vi "Actor Core.vi"(8 "error in":errorcluster, 11 "CS++ScopeGui.lvclass":refnum<class "CS++ScopeGui.lvclass">) -> (0 "Error Out":errorcluster, 3 "Actor out":refnum<class "Actor.lvclass">)   [LabVIEW 2015, in "CS++ScopeGui.lvlib" / "CS++ScopeGui.lvclass"]
doc: "(<B>Filename</B>: Actor Framework.lvlib:Actor.lvclass:Actor Core.vi)\n\nReceives messages to the actor, reacts to them, and initiates any error handling that may shut the actor down.\n\nDescendant classes may override this VI to append parallel tasks for the actor to complete while it handles messages. Overrides use the Call Parent Method node."
uses:
  CS++ScopeGui.lvclass
  <vilib>/ActorFramework/Actor/Actor.lvclass
  CSPP_Core/Actors/CS++BaseActor/CS++BaseActor.lvclass/CS++BaseActor.ctl
  CSPP_Core/Actors/CS++GUIActor/CS++GUIActor.lvclass/CS++GUIActor.ctl
  CSPP_Core/Classes/CS++ProcessVariables/ProcessVariable/PV.lvclass/PV.ctl
  <vilib>/ActorFramework/Actor/Actor.lvclass/Actor.ctl
  <vilib>/ActorFramework/Message Enqueuer/Message Enqueuer.lvclass/Message Enqueuer.ctl
  CSPP_Core/Actors/CS++BaseActor/Read Object Name.vi
  CSPP_Core/Actors/CS++BaseActor/Read CS++Factory.vi
  CSPP_Core/Actors/CS++GUIActor/Read Associated Actor Name.vi
  CSPP_Core/Classes/CS++ProcessVariables/ProcessVariable/Read Data.vi
  CSPP_Core/Classes/CS++ProcessVariables/ProcessVariable/Read Timestamp.vi
  CSPP_Core/Classes/CS++ProcessVariables/ProcessVariable/Read Name.vi
  CSPP_Core/Actors/CS++GUIActor/Read Stop-Event.vi
  CSPP_Core/Actors/CS++GUIActor/Read PV-Update.vi
  CSPP_Core/Actors/CS++GUIActor/Read Associated Proxy Actor Enqueuer.vi
  <vilib>/ActorFramework/Message Enqueuer/Init from Existing Queue.vi
  <vilib>/ActorFramework/Message Enqueuer/Enqueue.vi
  <vilib>/Utility/file.llb/Write To Spreadsheet File (DBL).vi
  <vilib>/ActorFramework/Message Priority Queue/Priority Enqueue.vi
  CSPP_Core/Classes/CS++ProcessVariables/PVConnection/PVConnection.lvclass
  CSPP_Core/Classes/CS++BaseClasses/Factory/CS++Factory.lvclass
  CSPP_Core/Classes/CS++ProcessVariables/ProcessVariable/PV.lvclass
  <vilib>/ActorFramework/Message Enqueuer/Message Enqueuer.lvclass
  <vilib>/ActorFramework/Stop Msg/Stop Msg.lvclass
  CSPP_Core/Actors/CS++DeviceGUIActor/CS++DeviceGUIActor.lvclass
  CSPP_Core/Libraries/Utilities/CS++Utilities.lvlib
  CSPP_Core/Actors/CS++BaseActor/CS++BaseActor.lvclass
  CSPP_Core/Actors/CS++GUIActor/CS++GUIActor.lvclass
panel:
  out "Channel Enabled?":bool[](array[boolean])
  in  "NotFirstStart":bool
  in  "OrgCurPosRight":dbl=0.4
  in  "OrgCurPosLeft":dbl=-0.4
  in  "LHS":i16=23
  in  "OrigCursPosVer":dbl[](array[numeric])=[1.25, -1.25]
  in  "DatCount":i32
  in  "Start":bool
  in  "LastModGraph":i8
  in  "Scaling-Array":dbl[](array[numeric])=[1.0, 1.0, 1.0, 1.0]
  out "LastHorOffset":dbl
  out "Complete\nData":cluster{"Array":dbl[], "Y":dbl[]}[](array[cluster])
  out "Time/Record":dbl
  out "size(s)":i32
  out "x-y":dbl
  in  "Tab Control":enum32{"Info", "Measurement"}(tab)
  out "Last Update":timestamp
  out "Associated Device Actor":string
  out "Resource Name":string
  out "Self-Test Result Message":string
  out "Self-Test Result Code":i32
  out "Firmware Revision":string
  out "Driver Revision":string
  in  "Trigger Slope":u16(ring) caption="Source" items=["Rising", "Falling"]
  in  "Trigger Source":u16(ring) caption="Source"
  in  "Trigger Level":dbl[unit] caption="Level"
  in  "One Button":bool
  in  "Abort Button":bool
  in  "RepeatButton":bool
  out "Scope Graph":cluster{dbl[], "Y":dbl[]}[](graph)
  in  "Status LED":u32(colorbox)
  in  "Config Table":string[][](table)=[["DC", "DC", "DC", "DC"], ["2", "2", "2", "2"], ["0", "0", "0", "0"], ["1", "1", "1", "1"]]
  out "Time / DIV":dbl[unit]=0.1
  in  "Horizontal Scale":i16(knob)=23 scale=0.0..31.0
  in  "Horizontal Offset":dbl[unit]
  # "Trigger"
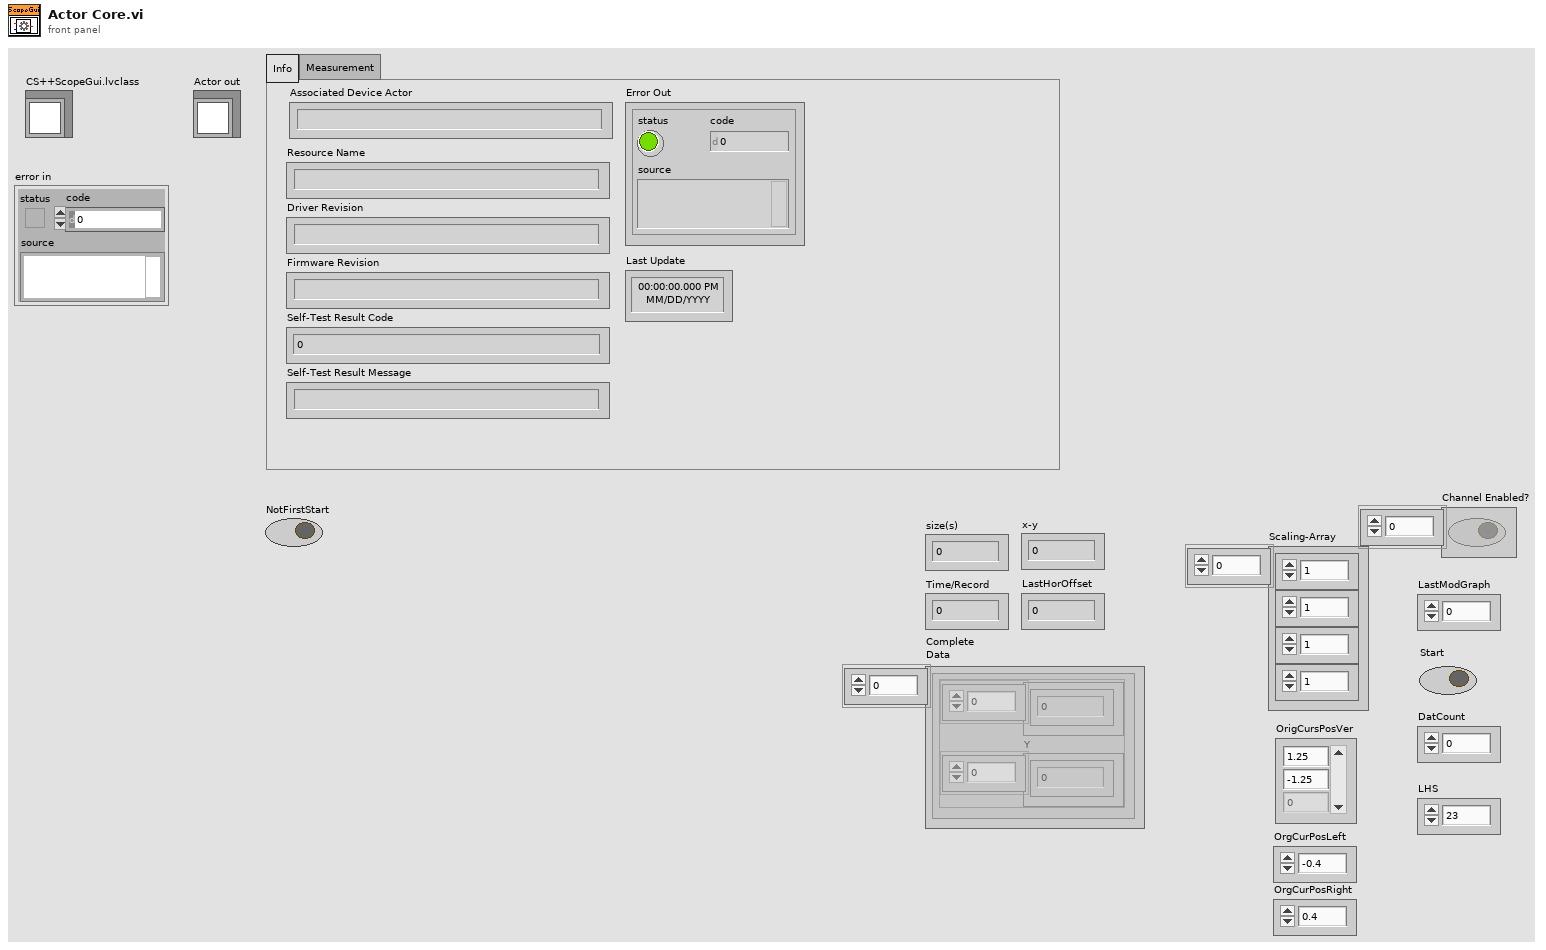
[diagram p1: front panel]
types:
  T1 = enum32{"Invalid", "Standard", "Closed", "Hidden", "Minimized", "Maximized"}
  T2 = typedef "LVAnnotationListTypeDef.ctl" = cluster{"Name":string, "Color":u32, "Style":u8, "Point Style":u8, "Name Visible":bool, "Allow Drag":bool, "Annotation Mode":u32, "Plot":i32, "Index":i32, "Position":cluster{"X":dbl, "Y":dbl}, "X Scale":u32, "Y Scale":u32, "Show Arrow":bool, "Lock Name":bool, "Plot Area":i32, "Label Offset":cluster{"X":dbl, "Y":dbl}}[]
  T3 = cluster{"Name":string, "Color":u32, "Style":u8, "Point Style":u8, "Name Visible":bool, "Allow Drag":bool, "Annotation Mode":u32, "Plot":i32, "Index":i32, "Position":cluster{"X":dbl, "Y":dbl}, "X Scale":u32, "Y Scale":u32, "Show Arrow":bool, "Lock Name":bool, "Plot Area":i32, "Label Offset":cluster{"X":dbl, "Y":dbl}}
  T4 = cluster{"Substring":string, dbl, dbl[unit], dbl[unit], bool, "vertical coupling (DC)":i32}
  T5 = cluster{dbl[unit], "min record length (100 samples)":i32, dbl[unit]}
  T6 = cluster{"Substring":string, "Trigger Level":dbl[unit], i16}
  T7 = cluster{"Substring":string, "NewVal":dbl[unit], i16}
  T8 = cluster{"Substring":string, dbl, dbl[unit], dbl[unit], "Plot.Visible?":bool, "vertical coupling (DC)":i32}
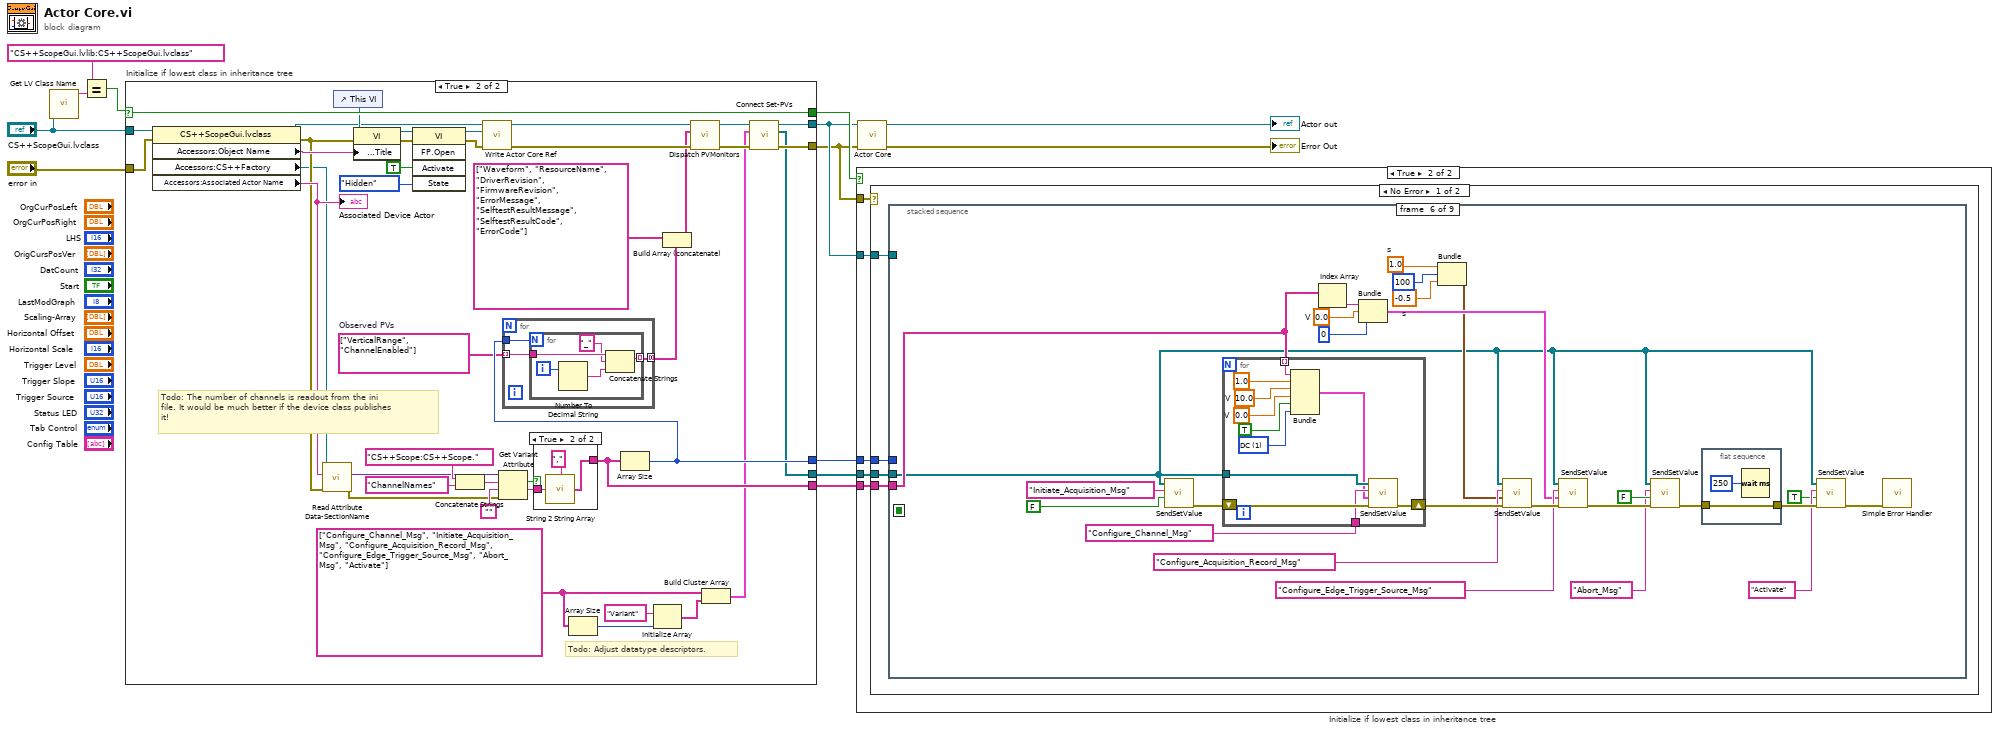
[diagram p0: block diagram]
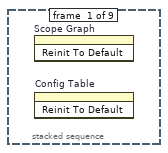
[diagram p5: hidden frame]
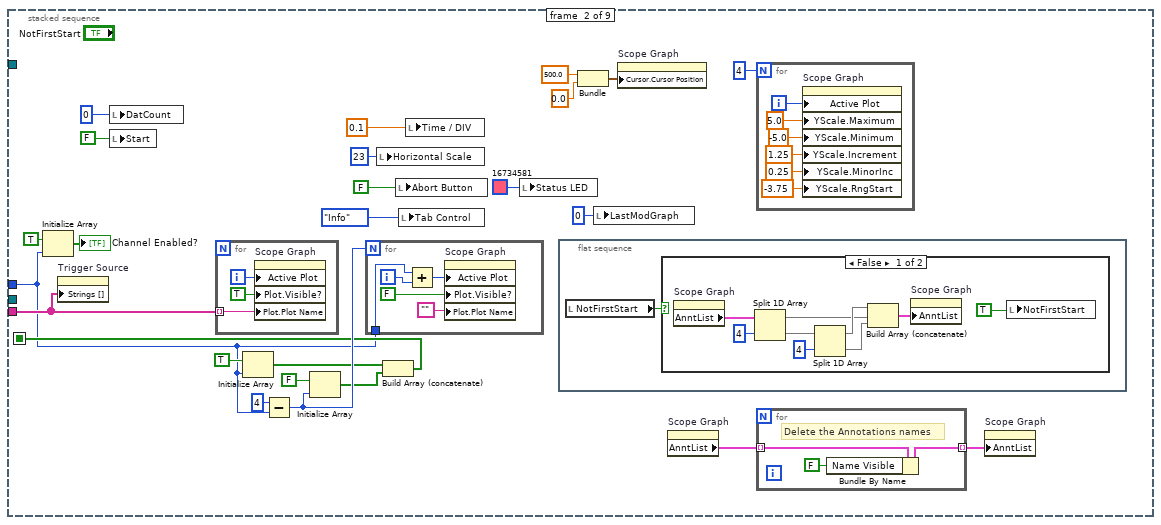
[diagram p6: hidden frame]
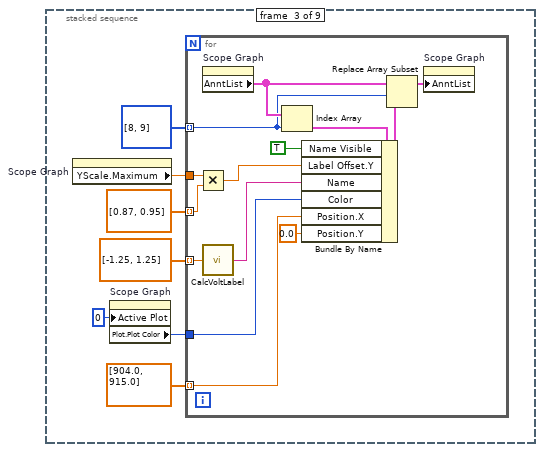
[diagram p8: hidden frame]
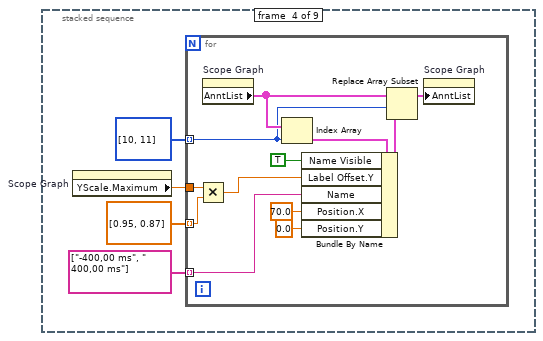
[diagram p9: hidden frame]
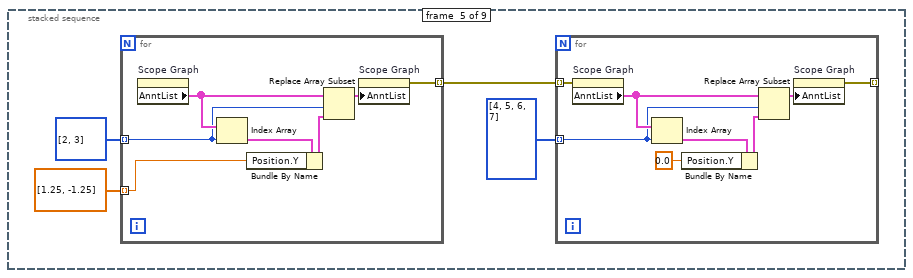
[diagram p10: hidden frame]
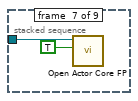
[diagram p11: hidden frame]
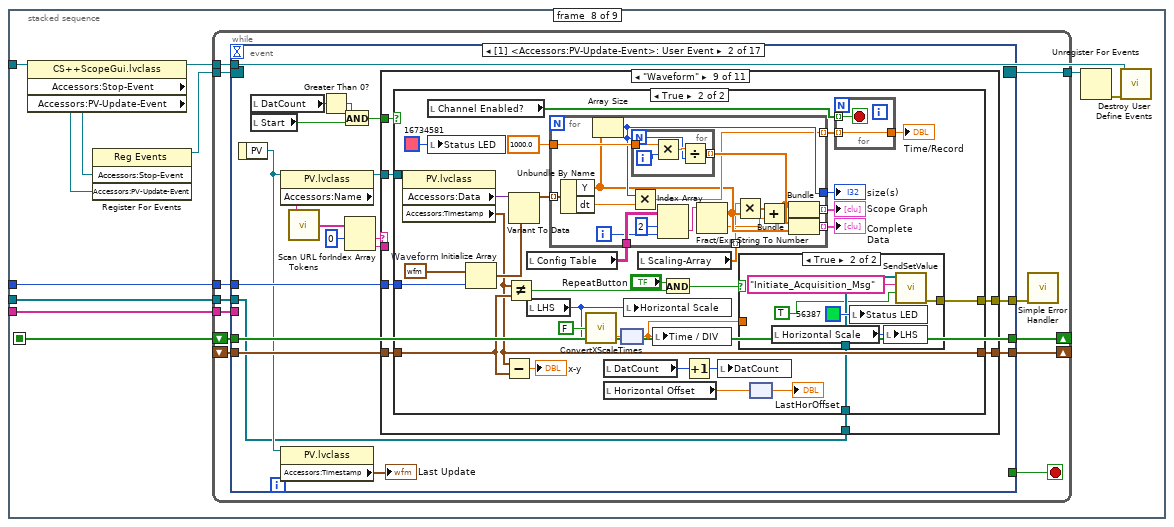
[diagram p12: hidden frame]
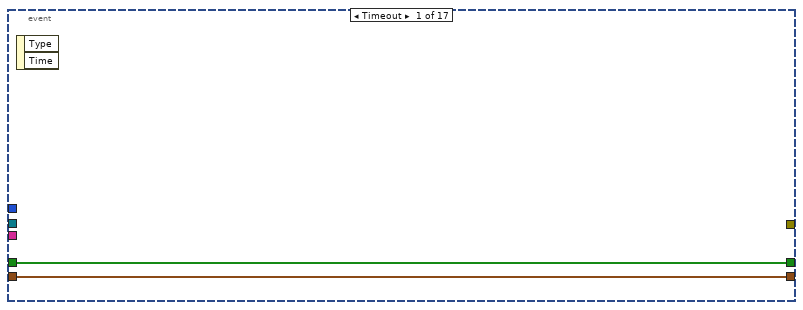
[diagram p13: hidden frame]
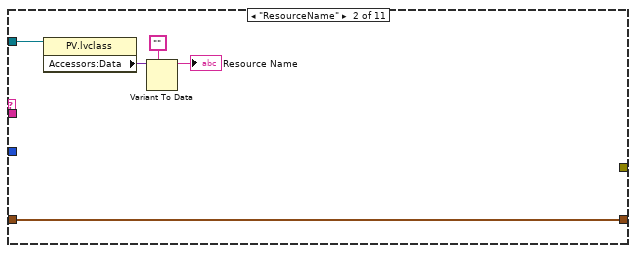
[diagram p15: hidden frame]
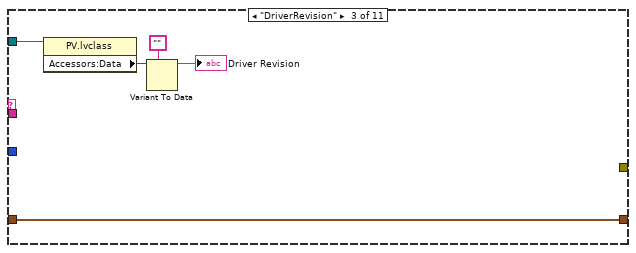
[diagram p16: hidden frame]
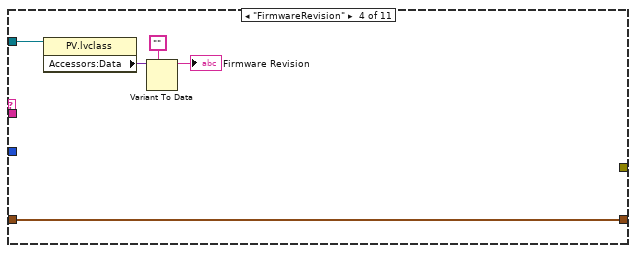
[diagram p17: hidden frame]
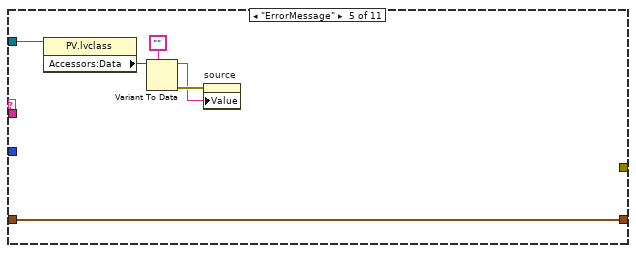
[diagram p18: hidden frame]
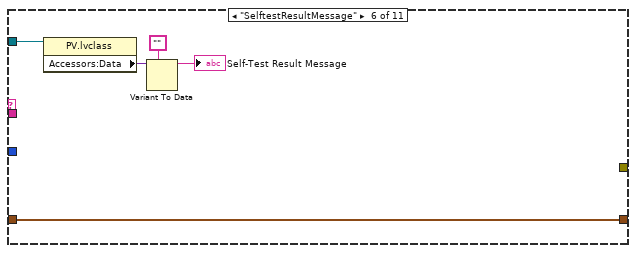
[diagram p19: hidden frame]
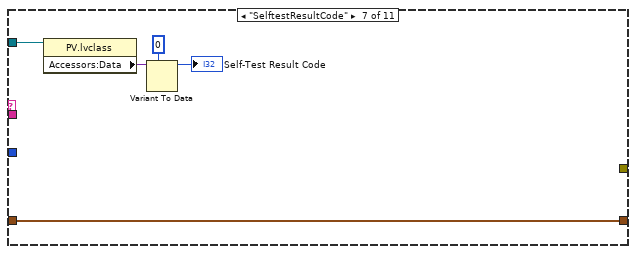
[diagram p20: hidden frame]
diagram:
  n1 = call <vilib>:"Get LV Class Name.vi"("object"="CS++ScopeGui.lvclass") -> ("class name"=w11:string)  [unwired: 9 in, 1 out]
  n2 = Equal?(x="CS++ScopeGui.lvlib:CS++ScopeGui.lvclass" ("class name"), y=w11) -> (x = y?=w9:bool)
  n3 = case "Initialize if lowest class in inheritance tree" shown="True" w9 {
    selector: w9 -> [w14 w57]
    tunnel: [w15 w24] -> w5
    tunnel: "error in" -> [w15 w37]
    tunnel: [w16 w25] -> w6
    tunnel: "CS++ScopeGui.lvclass" -> [w16 w38]
    tunnel: [w14 w57] -> w8
    tunnel: [_ w32] -> w3
    tunnel: [_ w50] -> w2
    tunnel: [_ w22] -> w1
    frame False {
    }
    frame True {
      w21 = string[] ["Configure_Channel_Msg", "Initiate_Acquisition_Msg", "Configure_Acquisition_Record_Msg", "Configure_Edge_Trigger_Source_Msg", "Abort_Msg", "Activate"]
      w31 = string[] ["VerticalRange", "ChannelEnabled"]  # Observed PVs
      # "Todo: Adjust datatype descriptors."
      # "Todo: The number of channels is readout from the ini\nfile. It would be much better if the device class publishes\nit!"
      n4 = property class="CS++ScopeGui.lvclass"(reference=w38, error in=w37) -> (reference out=w42:refnum<class "CS++ScopeGui.lvclass">, error out=w35:errorcluster, "Accessors:Object Name"=w41:string, "Accessors:CS++Factory"=w27:refnum<class "CS++Factory.lvclass">, "Accessors:Associated Actor Name"=w36:string)
      "Associated Device Actor" <- w36
      n5 = call-dynamic "Read Attribute Data-SectionName.vi"("error in (no error)"=w35, "Object Name"=w36, "CS++Factory in"=w27) -> ("error out"=w33:errorcluster, "Attribute Data"=w34:variant)  [unwired: 6 in, 1 out]
      n6 = control-ref of="This VI"() -> (w45:refnum<vi>)
      n7 = property class="VI"(reference=w45, error in=w35, "Front Panel.Title"=w41) -> (reference out=w44:refnum<vi>, error out=w43:errorcluster)
      n8 = invoke class="VI" method="FP.Open"(reference=w44, error in=w43, "Activate"=TRUE ("Activate?"), "State"=T1."Hidden") -> (reference out=w47:refnum<vi>, error out=w46:errorcluster)  [unwired: 1 in, 3 out]
      n9 = Concatenate Strings("CS++Scope:CS++Scope.", "ChannelNames" ("string")) -> (w55:string)
      n10 = call "Write Actor Core Ref.vi"("error in (no error)"=w46, "Actor Core Ref"=w47, "CS++BaseActor in"=w42) -> ("error out"=w39:errorcluster, "CS++BaseActor out"=w40:refnum<class "CS++ScopeGui.lvclass">)  [unwired: 7 in]
      n11 = Get Variant Attribute(Variant=w34, name=w55, default value (empty Variant)="", error in=w33) -> (found=w52:bool, value=w53:string)  [unwired: 2 out]
      n12 = case shown="True" w52 {
        tunnel: w53 -> [_ w68]
        tunnel: [_ w66] -> w50
        frame False {
        }
        frame True {
          n13 = call "String 2 String Array.vi"("String"=w68, "Delimiter (\",\")"="," ("Delimiter (\",\")")) -> ("Substrings"=w66:string[])
        }
      }
      n14 = Array Size(array=w21) -> (size(s)=w20:i32)
      n15 = Array Size(array=w50) -> (size(s)=w32:i32)
      n16 = for {
        tunnel: w32 -> [w60]
        tunnel: w31 -> [w59] mode=indexing
        tunnel: [w58] -> w30 mode=concatenating
        n17 = for {
          N: w60 -> [_]
          tunnel: w59 -> [w65]
          tunnel: [w64] -> w58 mode=indexing
          i -> [w63]
          n18 = Number To Decimal String(number=w63) -> (decimal integer string=w62:string)  [unwired: 1 in]
          n19 = Concatenate Strings(w65, "_" ("string"), w62) -> (w64:string)
        }
      }
      n20 = Initialize Array("Variant", w20) -> (w17:string[])
      n21 = Build Array (concatenate)(string[] ["Waveform", "ResourceName", "DriverRevision", "FirmwareRevision", "ErrorMessage", "SelftestResultMessage", "SelftestResultCode", "ErrorCode"], w30) -> (w29:string[])
      n22 = call "Dispatch PVMonitors.vi"("Error In"=w39, "PV Names (empty)"=w29, "CS++GUIActor in"=w40) -> ("Error Out"=w23:errorcluster, "CS++GUIActor out"=w26:refnum<class "CS++ScopeGui.lvclass">)  [unwired: 7 in]
      n23 = Build Cluster Array(w21, w17) -> (w18:cluster{string, string}[])
      n24 = call "Connect Set-PVs.vi"("Error In"=w23, "Set-Messages"=w18, "CS++GUIActor in"=w26) -> ("Error Out"=w24:errorcluster, "PVConnections"=w22:refnum<class "PVConnection.lvclass">[], "CS++GUIActor out"=w25:refnum<class "CS++ScopeGui.lvclass">)  [unwired: 6 in]
    }
  }
  n25 = case "Initialize if lowest class in inheritance tree" shown="True" w8 {
    tunnel: w5 -> [_ w73]
    tunnel: w6 -> [_ w72]
    tunnel: w3 -> [_ w71]
    tunnel: w2 -> [_ w70]
    tunnel: w1 -> [_ w69]
    frame False {
    }
    frame True {
      n26 = case shown="No Error" w73 {
        tunnel: w72 -> [w77 _]
        tunnel: w71 -> [w76 _]
        tunnel: w70 -> [w75 _]
        tunnel: w69 -> [w74 _]
        frame No Error {
          n27 = stacked-sequence {
            seq-local: [_ w86 _ _ _ _ _ _ _] -> [_ _ _ _ _ _ _ w235 _]
            tunnel: w77 -> [_ _ _ _ _ _ w225 w232 w1117]
            tunnel: w76 -> [_ w79 _ _ _ _ _ w237 _]
            tunnel: w75 -> [_ w93 _ _ _ w200 _ w236 _]
            tunnel: w74 -> [_ _ _ _ _ w188 _ w227 w1115]
            frame #0 {
              n28 = invoke on="Scope Graph" class="XYGraph (strict)" method="Reinit To Default"() -> ()  [unwired: 3 in, 3 out]
              n29 = invoke on="Config Table" class="Tbl (strict)" method="Reinit To Default"() -> ()  [unwired: 3 in, 3 out]
            }
            frame #1 {
              n30 = Initialize Array(TRUE ("Open FP (F)"), w79) -> (→"Channel Enabled?":bool[])
              n31 = property on="Trigger Source" class="Ring (strict)"("Strings []"=w93) -> ()  [unwired: 2 in, 2 out]
              n32 = local write "DatCount"(0 ("DataCounter")) -> ()
              n33 = local write "Start"(FALSE ("Start")) -> ()
              n34 = for {
                tunnel: w93 -> [w127] mode=indexing
                i -> [w129]
                n35 = property on="Scope Graph" class="XYGraph (strict)"("Active Plot"=w129, "Plot.Visible?"=TRUE ("Plot.Visible"), "Plot.Plot Name"=w127) -> ()  [unwired: 2 in, 2 out]
              }
              n36 = Initialize Array(TRUE ("Plot.Visible?"), w79) -> (w88:bool[])
              n37 = Subtract(x=4, y=w79) -> (x-y=w89:i32)
              n38 = Initialize Array(FALSE ("Plot.Visible?"), w89) -> (w87:bool[])
              n39 = for {
                N: w89 -> [_]
                tunnel: w79 -> [w120]
                i -> [w122]
                n40 = Add(x=w120, y=w122) -> (x+y=w121:i32)
                n41 = property on="Scope Graph" class="XYGraph (strict)"("Active Plot"=w121, "Plot.Visible?"=FALSE ("Plot.Visible"), "Plot.Plot Name"="") -> ()  [unwired: 2 in, 2 out]
              }
              n42 = local write "Horizontal Scale"(i16 23 ("Horizontal Scale")) -> ()
              n43 = Build Array (concatenate)(w88, w87) -> (w86:bool[])
              n44 = local write "Abort Button"(FALSE ("Stop Button")) -> ()
              n45 = local write "Tab Control"(enum32{"Info", "Measurement"}."Info" ("Tab Control")) -> ()
              n46 = local write "Time / DIV"(dbl[unit] 0.1 ("Time / DIV")) -> ()
              n47 = local write "Status LED"(u32 16734581) -> ()
              n48 = flat-sequence {
                frame #0 {
                  n49 = local read "NotFirstStart"() -> (w103:bool)
                  n50 = case shown="False" w103 {
                    frame False {
                      n51 = property on="Scope Graph" class="XYGraph (strict)"() -> ("AnntList"=w112:T2)  [unwired: 2 in, 2 out]
                      n52 = Split 1D Array(array=w112, index=4) -> (first subarray=w107:T2, second subarray=w110:T2)
                      n53 = Split 1D Array(array=w110, index=4) -> (first subarray=w108:T2, second subarray=w106:T2)
                      n54 = Build Array (concatenate)(w108, w107, w106) -> (w105:T2)
                      n55 = property on="Scope Graph" class="XYGraph (strict)"("AnntList"=w105) -> ()  [unwired: 2 in, 2 out]
                      n56 = local write "NotFirstStart"(TRUE ("FirstStart")) -> ()
                    }
                    frame True {
                    }
                  }
                }
              }
              n57 = Bundle(500.0, 0.0) -> (w94:cluster{dbl, dbl})  [unwired: 1 in]
              n58 = local write "LastModGraph"(u8 0 ("LastModifiedGraph")) -> ()
              n59 = property on="Scope Graph" class="XYGraph (strict)"("Cursor.Cursor Position"=w94) -> ()  [unwired: 2 in, 2 out]
              n60 = property on="Scope Graph" class="XYGraph (strict)"() -> ("AnntList"=w100:T2)  [unwired: 2 in, 2 out]
              n61 = for {
                N: 4 -> [_]
                i -> [w118]
                n62 = property on="Scope Graph" class="XYGraph (strict)"("Active Plot"=w118, "YScale.Maximum"=5.0, "YScale.Minimum"=-5.0 ("Y Scale.Range:Minimum"), "YScale.Increment"=1.25 ("Y Scale.Range:Increment"), "YScale.MinorInc"=0.25 ("Y Scale.Range:Minor Increment"), "YScale.RngStart"=-3.75 ("Y Scale.Range:Start")) -> ()  [unwired: 2 in, 2 out]
              }
              n63 = for {
                tunnel: w100 -> [w125] mode=indexing
                tunnel: [w124] -> w99 mode=indexing
                # "Delete the Annotations names"
                n64 = Bundle By Name(cluster=w125, "Name Visible"=FALSE) -> (w124:T3)
              }
              n65 = property on="Scope Graph" class="XYGraph (strict)"("AnntList"=w99) -> ()  [unwired: 2 in, 2 out]
            }
            frame #2 {
              n66 = property on="Scope Graph" class="XYGraph (strict)"() -> ("YScale.Maximum"=w135:dbl)  [unwired: 2 in, 2 out]
              n67 = property on="Scope Graph" class="XYGraph (strict)"("Active Plot"=u32 0) -> ("Plot.Plot Color"=w132:u32)  [unwired: 2 in, 2 out]
              n68 = for {
                tunnel: i32[] [8, 9] -> [w145] mode=indexing
                tunnel: w135 -> [w143]
                tunnel: dbl[] [0.87, 0.95] -> [w142] mode=indexing
                tunnel: dbl[] [-1.25, 1.25] -> [w138] mode=indexing
                tunnel: w132 -> [w141]
                tunnel: dbl[] [904.0, 915.0] -> [w140] mode=indexing
                n69 = Multiply(x=w143, y=w142) -> (x*y=w144:dbl)
                n70 = property on="Scope Graph" class="XYGraph (strict)"() -> ("AnntList"=w149:T2)  [unwired: 2 in, 2 out]
                n71 = call "CalcVoltLabel.vi"("InputVolt"=w138) -> ("VoltString"=w137:string)
                n72 = Index Array(array=w149, index=w145) -> (element=w148:T3)
                n73 = Bundle By Name(cluster=w148, "Name Visible"=TRUE, "Label Offset.Y"=w144, "Name"=w137, "Color"=w141, "Position.X"=w140, "Position.Y"=0.0) -> (w147:T3)
                n74 = Replace Array Subset(array=w149, new element=w147, index=w145) -> (w150:T2)
                n75 = property on="Scope Graph" class="XYGraph (strict)"("AnntList"=w150) -> ()  [unwired: 2 in, 2 out]
              }
            }
            frame #3 {
              n76 = property on="Scope Graph" class="XYGraph (strict)"() -> ("YScale.Maximum"=w153:dbl)  [unwired: 2 in, 2 out]
              n77 = for {
                tunnel: i32[] [10, 11] -> [w161] mode=indexing
                tunnel: w153 -> [w159]
                tunnel: dbl[] [0.95, 0.87] -> [w158] mode=indexing
                tunnel: string[] ["-400,00 ms", " 400,00 ms"] -> [w157] mode=indexing
                n78 = Multiply(x=w159, y=w158) -> (x*y=w160:dbl)
                n79 = property on="Scope Graph" class="XYGraph (strict)"() -> ("AnntList"=w165:T2)  [unwired: 2 in, 2 out]
                n80 = Index Array(array=w165, index=w161) -> (element=w164:T3)
                n81 = Bundle By Name(cluster=w164, "Name Visible"=TRUE, "Label Offset.Y"=w160, "Name"=w157, "Position.X"=70.0, "Position.Y"=0.0) -> (w163:T3)
                n82 = Replace Array Subset(array=w165, new element=w163, index=w161) -> (w166:T2)
                n83 = property on="Scope Graph" class="XYGraph (strict)"("AnntList"=w166) -> ()  [unwired: 2 in, 2 out]
              }
            }
            frame #4 {
              n84 = for {
                tunnel: i32[] [2, 3] -> [w181] mode=indexing
                tunnel: dbl[] [1.25, -1.25] -> [w180] mode=indexing
                tunnel: [w179] -> w168 mode=indexing
                n85 = property on="Scope Graph" class="XYGraph (strict)"() -> ("AnntList"=w184:T2)  [unwired: 2 in, 2 out]
                n86 = Index Array(array=w184, index=w181) -> (element=w183:T3)
                n87 = Bundle By Name(cluster=w183, "Position.Y"=w180) -> (w182:T3)
                n88 = Replace Array Subset(array=w184, new element=w182, index=w181) -> (w185:T2)
                n89 = property on="Scope Graph" class="XYGraph (strict)"("AnntList"=w185) -> (error out=w179:errorcluster)  [unwired: 2 in, 1 out]
              }
              n90 = for {
                tunnel: i32[] [4, 5, 6, 7] -> [w174] mode=indexing
                tunnel: [w173] -> _ mode=indexing
                tunnel: w168 -> [w172] mode=indexing
                n91 = property on="Scope Graph" class="XYGraph (strict)"(error in=w172) -> ("AnntList"=w177:T2)  [unwired: 1 in, 2 out]
                n92 = Index Array(array=w177, index=w174) -> (element=w176:T3)
                n93 = Bundle By Name(cluster=w176, "Position.Y"=0.0) -> (w175:T3)
                n94 = Replace Array Subset(array=w177, new element=w175, index=w174) -> (w178:T2)
                n95 = property on="Scope Graph" class="XYGraph (strict)"("AnntList"=w178) -> (error out=w173:errorcluster)  [unwired: 2 in, 1 out]
              }
            }
            frame #5 {
              w196 = dbl[unit] -0.5  # s
              w198 = dbl[unit] 1.0  # s
              w202 = dbl[unit] 0.0  # V
              n96 = call "SendSetValue.vi"("Data"=FALSE, "PVName"="Initiate_Acquisition_Msg", "PVConnections"=w188) -> ("error out"=w209:errorcluster)  [unwired: 7 in, 1 out]
              n97 = for {
                tunnel: w188 -> [w222]
                tunnel: "Configure_Channel_Msg" -> [w221]
                shift-right: [w223] -> w208
                shift-left: w209 -> [w224]
                tunnel: w200 -> [w217] mode=indexing
                w214 = dbl[unit] 0.0  # V
                w215 = dbl[unit] 10.0  # V
                w220 = 1 items=["AC", "DC", "GND"] ("vertical coupling (DC)")
                n98 = Bundle("Substring"=w217, 1.0, w215, w214, TRUE, "vertical coupling (DC)"=w220) -> (w218:T4)  [unwired: 1 in]
                n99 = call "SendSetValue.vi"("error in (no error)"=w224, "Data"=w218, "PVName"=w221, "PVConnections"=w222) -> ("error out"=w223:errorcluster)  [unwired: 6 in, 1 out]
              }
              n100 = Index Array(array=w200) -> (element=w201:string)  [unwired: 1 in]
              n101 = Bundle("Substring"=w201, w202, i16 0) -> (w199:cluster{"Substring":string, dbl[unit], i16})  [unwired: 1 in]
              n102 = Bundle(w198, "min record length (100 samples)"=100, w196) -> (w197:T5)  [unwired: 1 in]
              n103 = call "SendSetValue.vi"("error in (no error)"=w208, "Data"=w197, "PVName"="Configure_Acquisition_Record_Msg", "PVConnections"=w188) -> ("error out"=w207:errorcluster)  [unwired: 6 in, 1 out]
              n104 = call "SendSetValue.vi"("error in (no error)"=w207, "Data"=w199, "PVName"="Configure_Edge_Trigger_Source_Msg", "PVConnections"=w188) -> ("error out"=w190:errorcluster)  [unwired: 6 in, 1 out]
              n105 = call "SendSetValue.vi"("error in (no error)"=w190, "Data"=FALSE, "PVName"="Abort_Msg", "PVConnections"=w188) -> ("error out"=w189:errorcluster)  [unwired: 6 in, 1 out]
              n106 = flat-sequence {
                tunnel: [w213] -> w193
                tunnel: w189 -> [w213]
                frame #0 {
                  n107 = Wait (ms)(milliseconds to wait=u32 250) -> ()  [unwired: 1 out]
                }
              }
              n108 = call "SendSetValue.vi"("error in (no error)"=w193, "Data"=TRUE, "PVName"="Activate", "PVConnections"=w188) -> ("error out"=w194:errorcluster)  [unwired: 6 in, 1 out]
              n109 = call <vilib>:"Simple Error Handler.vi"("error in (no error)"=w194) -> ()  [unwired: 4 in, 5 out]
            }
            frame #6 {
              n110 = call "Open Actor Core FP.vi"("Open FP (F)"=TRUE, "CS++BaseActor in"=w225) -> ()  [unwired: 8 in, 2 out]
            }
            frame #7 {
              n111 = property class="CS++ScopeGui.lvclass"(reference=w232) -> (reference out=w231:refnum<class "CS++ScopeGui.lvclass">, "Accessors:Stop-Event"=w229:refnum<user-event>, "Accessors:PV-Update-Event"=w228:refnum<user-event>)  [unwired: 1 in, 1 out]
              n112 = register-events(w229, w228) -> (reference out=w230:refnum<event-registration>)  [unwired: 2 in, 1 out]
              n113 = while {
                tunnel: w230 -> [w249]
                tunnel: w231 -> [w248]
                tunnel: [w246] -> w234
                tunnel: w237 -> [w244]
                shift-right: [w243] -> _
                shift-left: _ -> [w242]
                tunnel: w236 -> [w241]
                shift-right: [w240] -> _
                shift-left: w235 -> [w239]
                tunnel: w227 -> [w238]
                stop <- w247 stop-if-true
                n114 = event shown="[1] <Accessors:PV-Update-Event>: User Event" {
                  selector: w249 -> [_ _ _ _ _ _ _ _ _ _ _ _ _ _ _ _ _]
                  dyn-events: [_ _ _ _ _ _ _ _ _ _ _ _ _ _ _ _ _] -> w246
                  timeout: _ -> [_ _ _ _ _ _ _ _ _ _ _ _ _ _ _ _ _]
                  tunnel: w248 -> [_ _ _ _ _ _ _ _ _ _ _ _ _ _ _ _ w1109]
                  tunnel: [_ _ _ _ _ _ _ _ _ _ _ _ _ w1067 w1094 _ _] -> w247
                  tunnel: [_ w266 _ _ _ _ _ w632 w758 w770 w804 _ _ _ _ w1097 _] -> w245
                  tunnel: w244 -> [_ w265 _ _ _ _ _ w624 _ _ w781 _ _ w1066 _ _ _]
                  tunnel: [w251 w264 w482 w555 w594 w606 w618 w634 w757 w769 w806 w943 w1064 w1069 w1095 w1100 w1108] -> w243
                  tunnel: w242 -> [w251 w263 w482 w555 w594 w606 w618 w634 w757 w769 w806 w943 w1064 w1069 w1095 w1100 w1108]
                  tunnel: w241 -> [_ _ _ _ w597 w609 w621 w631 _ _ w803 _ _ _ _ _ _]
                  tunnel: [w250 w261 w483 w556 w595 w607 w619 w623 w756 w768 w783 w940 w1065 w1070 w1093 w1099 w1106] -> w240
                  tunnel: w239 -> [w250 w261 w483 w556 w595 w607 w619 w626 w756 w768 w783 w940 w1065 w1070 w1093 w1099 w1106]
                  tunnel: w238 -> [_ w252 w442 w518 w587 w599 w611 w622 w755 w767 w780 _ _ _ _ w1098 _]
                  event Timeout {
                    n115 = event-data() -> ()  [unwired: 1 in, 2 out]
                  }
                  event User Event {
                    n116 = event-data() -> ("PV"=w254:refnum<class "PV.lvclass">)  [unwired: 1 in]
                    n117 = local read "DatCount"() -> (w260:i32)
                    n118 = local read "Start"() -> (w258:bool)
                    n119 = property class="PV.lvclass"(reference=w254) -> (reference out=w256:refnum<class "PV.lvclass">, "Accessors:Name"=w255:string)  [unwired: 1 in, 1 out]
                    n120 = property class="PV.lvclass"(reference=w254) -> ("Accessors:Timestamp"=→"Last Update":timestamp)  [unwired: 1 in, 2 out]
                    n121 = call "Scan URL for Tokens.vi"("URL"=w255) -> ("Tokens"=w268:string[])
                    n122 = Greater Than 0?(x=w260) -> (x > 0?=w259:bool)
                    n123 = And(x=w259, y=w258) -> (x .and. y?=w257:bool)
                    n124 = Index Array(array=w268, index #1=0 ("index")) -> (element #1=w267:string, element #2=w262:string)  [unwired: 1 in]
                    n125 = case shown="\"Waveform\"" w267 {
                      tunnel: w256 -> [_ w273 w278 w283 w289 w294 w299 w305 w314 w411 w420]
                      tunnel: [_ _ _ _ _ _ _ _ w313 _ _] -> w266
                      tunnel: w265 -> [_ _ _ _ _ _ _ _ w312 w380 _]
                      tunnel: [w270 w271 w276 w281 w286 w292 w297 w302 w310 w410 w419] -> w264
                      tunnel: w263 -> [w270 w271 w276 w281 w286 w292 w297 w302 w311 w410 w419]
                      tunnel: w262 -> [_ _ _ _ _ _ _ _ _ w395 w418]
                      tunnel: w257 -> [_ _ _ _ _ _ _ _ w309 _ _]
                      tunnel: w252 -> [_ _ _ _ _ _ _ _ w308 _ _]
                      frame Default {
                      }
                      frame "ResourceName" {
                        n126 = property class="PV.lvclass"(reference=w273) -> ("Accessors:Data"=w275:variant)  [unwired: 1 in, 2 out]
                        n127 = Variant To Data(type="", Variant=w275) -> (data=→"Resource Name":string)  [unwired: 1 in, 1 out]
                      }
                      frame "DriverRevision" {
                        n128 = property class="PV.lvclass"(reference=w278) -> ("Accessors:Data"=w280:variant)  [unwired: 1 in, 2 out]
                        n129 = Variant To Data(type="", Variant=w280) -> (data=→"Driver Revision":string)  [unwired: 1 in, 1 out]
                      }
                      frame "FirmwareRevision" {
                        n130 = property class="PV.lvclass"(reference=w283) -> ("Accessors:Data"=w285:variant)  [unwired: 1 in, 2 out]
                        n131 = Variant To Data(type="", Variant=w285) -> (data=→"Firmware Revision":string)  [unwired: 1 in, 1 out]
                      }
                      frame "ErrorMessage" {
                        n132 = property class="PV.lvclass"(reference=w289) -> ("Accessors:Data"=w291:variant)  [unwired: 1 in, 2 out]
                        n133 = Variant To Data(type="", Variant=w291) -> (data=w287:string, error out=w288:errorcluster)  [unwired: 1 in]
                        n134 = property on="source" class="Str"(error in=w288, "Value"=w287) -> ()  [unwired: 1 in, 2 out]
                      }
                      frame "SelftestResultMessage" {
                        n135 = property class="PV.lvclass"(reference=w294) -> ("Accessors:Data"=w296:variant)  [unwired: 1 in, 2 out]
                        n136 = Variant To Data(type="", Variant=w296) -> (data=→"Self-Test Result Message":string)  [unwired: 1 in, 1 out]
                      }
                      frame "SelftestResultCode" {
                        n137 = property class="PV.lvclass"(reference=w299) -> ("Accessors:Data"=w301:variant)  [unwired: 1 in, 2 out]
                        n138 = Variant To Data(type=0, Variant=w301) -> (data=→"Self-Test Result Code":i32)  [unwired: 1 in, 1 out]
                      }
                      frame "ErrorCode" {
                        n139 = property class="PV.lvclass"(reference=w305) -> ("Accessors:Data"=w307:variant)  [unwired: 1 in, 2 out]
                        n140 = Variant To Data(type=0, Variant=w307) -> (data=w303:i32, error out=w304:errorcluster)  [unwired: 1 in]
                        n141 = property on="code" class="DigNum (strict)"(error in=w304, "Value"=w303) -> ()  [unwired: 1 in, 2 out]
                      }
                      frame "Waveform" {
                        n142 = case shown="True" w309 {
                          tunnel: w314 -> [_ w349]
                          tunnel: [_ w346] -> w313
                          tunnel: w312 -> [_ w343]
                          tunnel: w311 -> [w317 w341]
                          tunnel: [w317 w338] -> w310
                          tunnel: w308 -> [_ w319]
                          frame False {
                            n143 = local read "DatCount"() -> (w315:i32)
                            n144 = Increment(x=w315) -> (x+1=w316:i32)
                            n145 = local write "DatCount"(w316) -> ()
                          }
                          frame True {
                            w345 = waveform(dbl) {"t0"=timestamp(0 s since 1904-01-01), "dt"=1.0, "Y"=[]}  # Waveform
                            n146 = property class="PV.lvclass"(reference=w349) -> ("Accessors:Data"=w348:variant, "Accessors:Timestamp"=w338:timestamp)  [unwired: 1 in, 2 out]
                            n147 = local read "Channel Enabled?"() -> (w321:bool[])
                            n148 = local write "Status LED"(u32 16734581) -> ()
                            n149 = Initialize Array(w345, w343) -> (w344:waveform(dbl)[])
                            n150 = Subtract(x=w338, y=w341) -> (x-y=→"x-y":dbl)
                            n151 = Not Equal?(x=w338, y=w341) -> (x != y?=w339:bool)
                            n152 = Variant To Data(type=w344, Variant=w348) -> (data=w335:waveform(dbl)[])  [unwired: 1 in, 1 out]
                            n153 = local read "Config Table"() -> (w330:string[][])
                            n154 = local read "LHS"() -> (w324:i16)
                            n155 = call "ConvertXScaleTimes.vi"("InputKnob"=w324, "Time2Knob?"=FALSE) -> ("OutputTime"=w326:dbl)  [unwired: 2 in, 1 out]
                            n156 = local read "DatCount"() -> (w327:i32)
                            n157 = local read "Horizontal Offset"() -> (w331:dbl[unit])
                            n158 = node(w326) -> (w323:dbl[unit])
                            n159 = local write "Horizontal Scale"(w324) -> ()
                            n160 = local read "Scaling-Array"() -> (w329:dbl[])
                            n161 = for {
                              tunnel: [w361] -> w322 mode=indexing
                              tunnel: [w363] -> w337
                              tunnel: 1000.0 -> [w368]
                              tunnel: w335 -> [w367] mode=indexing
                              tunnel: [w366] -> w334 mode=indexing
                              tunnel: [w365] -> w333 mode=indexing
                              tunnel: w330 -> [w360]
                              tunnel: w329 -> [w352] mode=indexing
                              i -> [w358]
                              n162 = Unbundle By Name(w367) -> ("Y"=w355:dbl[], "dt"=w362:dbl)
                              n163 = Array Size(array=w355) -> (size(s)=w363:i32)
                              n164 = Multiply(x=w363, y=w362) -> (x*y=w361:dbl)
                              n165 = for {
                                N: w363 -> [w371]
                                tunnel: w368 -> [w369]
                                tunnel: [w373] -> w364 mode=indexing
                                i -> [w370]
                                n166 = Multiply(x=w369, y=w370) -> (x*y=w372:dbl)
                                n167 = Divide(x=w372, y=w371) -> (x/y=w373:dbl)
                              }
                              n168 = Index Array(array=w360, index (row)=2, index (col)=w358) -> (element=w357:string)
                              n169 = Fract/Exp String To Number(string=w357) -> (number=w354:dbl)  [unwired: 3 in, 1 out]
                              n170 = Multiply(x=w352, y=w355) -> (x*y=w353:dbl[])
                              n171 = Add(x=w353, y=w354) -> (x+y=w356:dbl[])
                              n172 = Bundle(w364, w356) -> (w366:cluster{dbl[], dbl[]})  [unwired: 1 in]
                              n173 = Bundle(w364, "Y"=w355) -> (w365:cluster{dbl[], "Y":dbl[]})  [unwired: 1 in]
                            }
                            "Scope Graph" <- w334
                            "size(s)" <- w337
                            "Complete\nData" <- w333
                            n174 = local write "Time / DIV"(w323) -> ()
                            n175 = And(x="RepeatButton", y=w339) -> (x .and. y?=w340:bool)
                            n176 = Increment(x=w327) -> (x+1=w328:i32)
                            n177 = local write "DatCount"(w328) -> ()
                            n178 = case shown="True" w340 {
                              tunnel: [_ w377] -> w346
                              tunnel: w323 -> [_ _]
                              tunnel: w319 -> [_ w376]
                              frame False {
                              }
                              frame True {
                                n179 = local read "Horizontal Scale"() -> (w378:i16)
                                n180 = local write "Status LED"(u32 56387) -> ()
                                n181 = local write "LHS"(w378) -> ()
                                n182 = call "SendSetValue.vi"("Data"=TRUE, "PVName"="Initiate_Acquisition_Msg", "PVConnections"=w376) -> ("error out"=w377:errorcluster)  [unwired: 7 in, 1 out]
                              }
                            }
                            n183 = node(w331) -> (→"LastHorOffset":dbl)
                            n184 = for {
                              tunnel: w322 -> [w350] mode=indexing
                              tunnel: w321 -> [w351] mode=indexing
                              tunnel: [w350] -> w320
                              stop <- w351 stop-if-true
                            }
                            "Time/Record" <- w320
                          }
                        }
                      }
                      frame "VerticalRange" {
                        n185 = local read "Config Table"() -> (w390:string[][])
                        n186 = Decimal String To Number(string=w395) -> (number=w385:i32)  [unwired: 2 in, 1 out]
                        n187 = property class="PV.lvclass"(reference=w411) -> ("Accessors:Data"=w394:variant)  [unwired: 1 in, 2 out]
                        n188 = Index Array(array=w390, index (row)=1) -> (element=w392:string[])  [unwired: 1 in]
                        n189 = Variant To Data(type=0.0, Variant=w394) -> (data=w383:dbl)  [unwired: 1 in, 1 out]
                        n190 = Array Subset(array=w392, length=w380) -> (w391:string[])  [unwired: 1 in]
                        n191 = Fract/Exp String To Number(string=w391) -> (number=w387:dbl[])  [unwired: 3 in, 1 out]
                        n192 = Divide(x=w383, y=8.0) -> (x/y=w382:dbl)
                        n193 = Replace Array Subset(array=w387, new element=w382, index=w385) -> (w386:dbl[])
                        n194 = Array Max & Min(array=w386) -> (min value=w388:dbl)  [unwired: 3 out]
                        n195 = Divide(x=w388, y=w386) -> (x/y=w384:dbl[])
                        n196 = Multiply(x=w388, y=8.0) -> (x*y=w402:dbl)
                        n197 = Divide(x=w402, y=2.0) -> (x/y=w403:dbl)
                        n198 = local write "Scaling-Array"(w384) -> ()
                        n199 = Number To Fractional String(number=w382, precision (6)=i16 2) -> (F-format string=w399:string)  [unwired: 2 in]
                        n200 = Divide(x=w403, y=4.0) -> (x/y=w405:dbl)
                        n201 = Divide(x=w405, y=5.0) -> (x/y=w404:dbl)
                        n202 = Replace Array Subset(array=w390, new element=w399, index (row)=1 ("disabled index (row)"), index (col)=w385) -> (w396:string[][])
                        n203 = Negate(x=w403) -> (-x=w408:dbl)
                        n204 = property on="Scope Graph" class="XYGraph (strict)"("Active Plot"=u32 0, "YScale.Maximum"=w403, "YScale.Minimum"=w408, "YScale.Increment"=w405, "YScale.MinorInc"=w404) -> ()  [unwired: 2 in, 2 out]
                        n205 = local write "Config Table"(w396) -> ()
                      }
                      frame "ChannelEnabled" {
                        n206 = property class="PV.lvclass"(reference=w420) -> ("Accessors:Data"=w422:variant)  [unwired: 1 in, 2 out]
                        n207 = Decimal String To Number(string=w418) -> (number=w412:i32)  [unwired: 2 in, 1 out]
                        n208 = local read "Channel Enabled?"() -> (w415:bool[])
                        n209 = Variant To Data(type=TRUE, Variant=w422) -> (data=w413:bool)  [unwired: 1 in, 1 out]
                        n210 = property on="Scope Graph" class="XYGraph (strict)"("Active Plot"=w412, "Plot.Visible?"=w413) -> ()  [unwired: 2 in, 2 out]
                        n211 = case shown="True" w413 {
                          tunnel: [u32 13816530 u32 0] -> w417
                          tunnel: [u32 13816530 w437] -> w416
                          tunnel: w412 -> [_ w436]
                          frame False {
                          }
                          frame True {
                            n212 = property on="Scope Graph" class="XYGraph (strict)"("Active Plot"=w436) -> ("Plot.Plot Color"=w437:u32)  [unwired: 2 in, 2 out]
                          }
                        }
                        n213 = Replace Array Subset(array=w415, new element=w413, index=w412) -> (w414:bool[])
                        n214 = local write "Channel Enabled?"(w414) -> ()
                        n215 = flat-sequence {
                          tunnel: w417 -> [w429]
                          tunnel: w416 -> [w428]
                          tunnel: w412 -> [w423]
                          frame #0 {
                            n216 = for {
                              N: 4 -> [_]
                              tunnel: w429 -> [w433]
                              tunnel: w423 -> [w431]
                              i -> [w430]
                              n217 = Bundle(w430, w431) -> (w432:cluster{i32, i32})  [unwired: 1 in]
                              n218 = property on="Config Table" class="Tbl (strict)"("Active Cell"=w432, "CellFontColor"=w433) -> ()  [unwired: 2 in, 2 out]
                            }
                            n219 = Bundle(-1, w423) -> (w426:cluster{i32, i32})  [unwired: 1 in]
                            n220 = property on="Config Table" class="Tbl (strict)"("Active Cell"=w426, "CellFontColor"=w428) -> ()  [unwired: 2 in, 2 out]
                            n221 = Wait (ms)(milliseconds to wait=u32 10) -> ()  [unwired: 1 out]
                          }
                        }
                      }
                    }
                  }
                  event "Horizontal Scale": Value Change {
                    w464 = 100.0 ("y")
                    # "The idea here is that half of the points\nhave to occure before the trigger!"
                    n222 = event-data() -> ("NewVal"=w481:i16)  [unwired: 1 in]
                    n223 = local read "OrgCurPosLeft"() -> (w458:dbl)
                    n224 = local read "OrgCurPosRight"() -> (w459:dbl)
                    n225 = call "ConvertXScaleTimes.vi"("InputKnob"=w481, "Time2Knob?"=FALSE) -> ("OutputTime"=w454:dbl)  [unwired: 2 in, 1 out]
                    n226 = node(w454) -> (→"Time / DIV":dbl[unit])
                    n227 = local read "Horizontal Offset"() -> (w456:dbl[unit])
                    n228 = local read "Complete\nData"() -> (w474:cluster{"Array":dbl[], "Y":dbl[]}[])
                    n229 = local read "Time/Record"() -> (w472:dbl)
                    n230 = local read "LastHorOffset"() -> (w470:dbl)
                    n231 = Multiply(x=w454, y=10.0) -> (x*y=w469:dbl)
                    n232 = Multiply(x=w454, y=5.0) -> (x*y=w457:dbl)
                    n233 = Add(x=w457, y=w458) -> (x+y=w460:dbl)
                    n234 = Add(x=w457, y=w459) -> (x+y=w461:dbl)
                    n235 = Negate(x=w457) -> (-x=w475:dbl)
                    n236 = node(w469) -> (w440:dbl[unit])
                    n237 = node(w475) -> (w476:dbl[unit])
                    n238 = node(w456) -> (w455:dbl)
                    n239 = Subtract(x=w460, y=w455) -> (x-y=w462:dbl)
                    n240 = Subtract(x=w461, y=w455) -> (x-y=w463:dbl)
                    n241 = Multiply(x=w462, y=w464) -> (x*y=w465:dbl)
                    n242 = Multiply(x=w463, y=w464) -> (x*y=w466:dbl)
                    n243 = Add(x=w476, y=w456) -> (x+y=w444:dbl[unit])
                    n244 = Divide(x=w465, y=w454) -> (x/y=w446:dbl)
                    n245 = Divide(x=w466, y=w454) -> (x/y=w445:dbl)
                    n246 = Divide(x=w472, y=w469) -> (x/y=w471:dbl)
                    n247 = property on="Scope Graph" class="XYGraph (strict)"() -> ("AnntList"=w449:T2)  [unwired: 2 in, 2 out]
                    n248 = Bundle(w440, 100, w444) -> (w443:cluster{dbl[unit], i32, dbl[unit]})  [unwired: 1 in]
                    n249 = local read "Config Table"() -> (w468:string[][])
                    n250 = Index Array(array=w449) -> (element #1=w448:T3, element #2=w451:T3)  [unwired: 2 in]
                    n251 = local read "Scaling-Array"() -> (w467:dbl[])
                    n252 = for {
                      tunnel: w474 -> [w512] mode=indexing
                      tunnel: [w511] -> w473 mode=indexing
                      tunnel: w471 -> [w508]
                      tunnel: w470 -> [w503]
                      tunnel: w469 -> [w505]
                      tunnel: w455 -> [w502]
                      tunnel: w468 -> [w498]
                      tunnel: w467 -> [w488] mode=indexing
                      i -> [w490]
                      w506 = 500.0 ("y")
                      n253 = Unbundle(w512) -> ("Array"=w510:dbl[], "Y"=w493:dbl[])
                      n254 = Index Array(array=w498, index (row)=2, index (col)=w490) -> (element=w497:string)
                      n255 = Subtract(x=w510, y=w506) -> (x-y=w509:dbl[])
                      n256 = Subtract(x=w502, y=w503) -> (x-y=w504:dbl)
                      n257 = Multiply(x=w508, y=w509) -> (x*y=w507:dbl[])
                      n258 = Divide(x=w504, y=w505) -> (x/y=w501:dbl)
                      n259 = Fract/Exp String To Number(string=w497) -> (number=w491:dbl)  [unwired: 3 in, 1 out]
                      n260 = Add(x=w506, y=w507) -> (x+y=w496:dbl[])
                      n261 = Multiply(x=w501, y=1000.0) -> (x*y=w495:dbl)
                      n262 = Multiply(x=w493, y=w488) -> (x*y=w489:dbl[])
                      n263 = Add(x=w496, y=w495) -> (x+y=w494:dbl[])
                      n264 = Add(x=w491, y=w489) -> (x+y=w492:dbl[])
                      n265 = Bundle(w494, w492) -> (w511:cluster{dbl[], dbl[]})  [unwired: 1 in]
                    }
                    n266 = Bundle By Name(cluster=w448, "Position.X"=w446) -> (w447:T3)
                    n267 = Bundle By Name(cluster=w451, "Position.X"=w445) -> (w452:T3)
                    n268 = Replace Array Subset(array=w449, new element #1=w447, new element #2=w452, index #2=1) -> (w450:T2)  [unwired: 1 in]
                    n269 = property on="Scope Graph" class="XYGraph (strict)"("AnntList"=w450) -> ()  [unwired: 2 in, 2 out]
                    n270 = flat-sequence {
                      tunnel: w473 -> [w487]
                      tunnel: w443 -> [w486]
                      tunnel: w442 -> [w485]
                      tunnel: "Configure_Acquisition_Record_Msg" -> [w484]
                      frame #0 {
                        n271 = local write "Scope Graph"(w487) -> ()
                        n272 = call "SendSetValue.vi"("Data"=w486, "PVName"=w484, "PVConnections"=w485) -> ()  [unwired: 7 in, 2 out]
                      }
                    }
                  }
                  event "Horizontal Offset": Value Change {
                    w540 = 100.0 ("y")
                    n273 = event-data() -> ("NewVal"=w531:dbl[unit])  [unwired: 1 in]
                    n274 = local read "OrgCurPosLeft"() -> (w534:dbl)
                    n275 = local read "OrgCurPosRight"() -> (w535:dbl)
                    n276 = local read "Time/Record"() -> (w550:dbl)
                    n277 = local read "Complete\nData"() -> (w552:cluster{"Array":dbl[], "Y":dbl[]}[])
                    n278 = local read "LastHorOffset"() -> (w545:dbl)
                    n279 = local read "Time / DIV"() -> (w520:dbl[unit])
                    n280 = Multiply(x=w520, y=10.0) -> (x*y=w514:dbl[unit])
                    n281 = Multiply(x=w520, y=5.0) -> (x*y=w533:dbl[unit])
                    n282 = node(w533) -> (w532:dbl)
                    n283 = Add(x=w532, y=w534) -> (x+y=w536:dbl)
                    n284 = Add(x=w532, y=w535) -> (x+y=w537:dbl)
                    n285 = Negate(x=w533) -> (-x=w548:dbl[unit])
                    n286 = node(w531) -> (w530:dbl)
                    n287 = Subtract(x=w536, y=w530) -> (x-y=w538:dbl)
                    n288 = Subtract(x=w537, y=w530) -> (x-y=w539:dbl)
                    n289 = Multiply(x=w538, y=w540) -> (x*y=w541:dbl)
                    n290 = Multiply(x=w539, y=w540) -> (x*y=w542:dbl)
                    n291 = node(w531) -> (w546:dbl)
                    n292 = node(w514) -> (w547:dbl)
                    n293 = node(w520) -> (w521:dbl)
                    n294 = Add(x=w548, y=w531) -> (x+y=w516:dbl[unit])
                    n295 = Divide(x=w541, y=w521) -> (x/y=w522:dbl)
                    n296 = Divide(x=w542, y=w521) -> (x/y=w519:dbl)
                    n297 = Divide(x=w550, y=w547) -> (x/y=w549:dbl)
                    n298 = Bundle(w514, 100, w516) -> (w515:cluster{dbl[unit], i32, dbl[unit]})  [unwired: 1 in]
                    n299 = property on="Scope Graph" class="XYGraph (strict)"() -> ("AnntList"=w525:T2)  [unwired: 2 in, 2 out]
                    n300 = local read "Config Table"() -> (w544:string[][])
                    n301 = Index Array(array=w525) -> (element #1=w524:T3, element #2=w527:T3)  [unwired: 2 in]
                    n302 = local read "Scaling-Array"() -> (w543:dbl[])
                    n303 = for {
                      tunnel: w552 -> [w585] mode=indexing
                      tunnel: [w584] -> w551 mode=indexing
                      tunnel: w549 -> [w581]
                      tunnel: w546 -> [w577]
                      tunnel: w547 -> [w578]
                      tunnel: w545 -> [w575]
                      tunnel: w544 -> [w571]
                      tunnel: w543 -> [w561] mode=indexing
                      i -> [w563]
                      w579 = 500.0 ("y")
                      n304 = Unbundle(w585) -> ("Array"=w583:dbl[], "Y"=w566:dbl[])
                      n305 = Subtract(x=w583, y=w579) -> (x-y=w582:dbl[])
                      n306 = Subtract(x=w577, y=w575) -> (x-y=w576:dbl)
                      n307 = Index Array(array=w571, index (row)=2, index (col)=w563) -> (element=w570:string)
                      n308 = Multiply(x=w581, y=w582) -> (x*y=w580:dbl[])
                      n309 = Divide(x=w576, y=w578) -> (x/y=w574:dbl)
                      n310 = Fract/Exp String To Number(string=w570) -> (number=w564:dbl)  [unwired: 3 in, 1 out]
                      n311 = Add(x=w579, y=w580) -> (x+y=w569:dbl[])
                      n312 = Multiply(x=w574, y=1000.0) -> (x*y=w568:dbl)
                      n313 = Multiply(x=w561, y=w566) -> (x*y=w562:dbl[])
                      n314 = Add(x=w569, y=w568) -> (x+y=w567:dbl[])
                      n315 = Add(x=w564, y=w562) -> (x+y=w565:dbl[])
                      n316 = Bundle(w567, w565) -> (w584:cluster{dbl[], dbl[]})  [unwired: 1 in]
                    }
                    n317 = Bundle By Name(cluster=w524, "Position.X"=w522) -> (w523:T3)
                    n318 = Bundle By Name(cluster=w527, "Position.X"=w519) -> (w528:T3)
                    n319 = Replace Array Subset(array=w525, new element #1=w523, new element #2=w528, index #2=1) -> (w526:T2)  [unwired: 1 in]
                    n320 = property on="Scope Graph" class="XYGraph (strict)"("AnntList"=w526) -> ()  [unwired: 2 in, 2 out]
                    n321 = flat-sequence {
                      tunnel: w551 -> [w560]
                      tunnel: w518 -> [w559]
                      tunnel: "Configure_Acquisition_Record_Msg" -> [w558]
                      tunnel: w515 -> [w557]
                      frame #0 {
                        n322 = local write "Scope Graph"(w560) -> ()
                        n323 = call "SendSetValue.vi"("Data"=w557, "PVName"=w558, "PVConnections"=w559) -> ()  [unwired: 7 in, 2 out]
                      }
                    }
                  }
                  event "Trigger Source": Value Change {
                    n324 = event-data() -> ("NewVal"=w596:u16)  [unwired: 1 in]
                    n325 = local read "Trigger Level"() -> (w590:dbl[unit])
                    n326 = local read "Trigger Slope"() -> (w592:u16)
                    n327 = Index Array(array=w597, index=w596) -> (element=w591:string)
                    n328 = Equal To 0?(x=w592) -> (x = 0?=w593:bool)
                    n329 = Boolean To (0,1)(Boolean=w593) -> (0, 1=w589:i16)
                    n330 = Bundle("Substring"=w591, "Trigger Level"=w590, w589) -> (w588:T6)  [unwired: 1 in]
                    n331 = call "SendSetValue.vi"("Data"=w588, "PVName"="Configure_Edge_Trigger_Source_Msg", "PVConnections"=w587) -> ()  [unwired: 7 in, 2 out]
                  }
                  event "Trigger Slope": Value Change {
                    n332 = event-data() -> ("NewVal"=w604:u16)  [unwired: 1 in]
                    n333 = local read "Trigger Source"() -> (w608:u16)
                    n334 = local read "Trigger Level"() -> (w602:dbl[unit])
                    n335 = Equal To 0?(x=w604) -> (x = 0?=w605:bool)
                    n336 = Boolean To (0,1)(Boolean=w605) -> (0, 1=w601:i16)
                    n337 = Index Array(array=w609, index=w608) -> (element=w603:string)
                    n338 = Bundle("Substring"=w603, "Trigger Level"=w602, w601) -> (w600:T6)  [unwired: 1 in]
                    n339 = call "SendSetValue.vi"("Data"=w600, "PVName"="Configure_Edge_Trigger_Source_Msg", "PVConnections"=w599) -> ()  [unwired: 7 in, 2 out]
                  }
                  event "Trigger Level": Value Change {
                    n340 = event-data() -> ("NewVal"=w614:dbl[unit])  [unwired: 1 in]
                    n341 = local read "Trigger Slope"() -> (w616:u16)
                    n342 = local read "Trigger Source"() -> (w620:u16)
                    n343 = Equal To 0?(x=w616) -> (x = 0?=w617:bool)
                    n344 = Boolean To (0,1)(Boolean=w617) -> (0, 1=w613:i16)
                    n345 = Index Array(array=w621, index=w620) -> (element=w615:string)
                    n346 = Bundle("Substring"=w615, "NewVal"=w614, w613) -> (w612:T7)  [unwired: 1 in]
                    n347 = call "SendSetValue.vi"("Data"=w612, "PVName"="Configure_Edge_Trigger_Source_Msg", "PVConnections"=w611) -> ()  [unwired: 7 in, 2 out]
                  }
                  event "Scope Graph": Plot Attribute Change {
                    n348 = event-data() -> ()  [unwired: 1 in, 1 out]
                    n349 = Subtract(x=4, y=w624) -> (x-y=w628:i32)
                    n350 = local read "Config Table"() -> (w630:string[][])
                    n351 = for {
                      N: w628 -> [_]
                      i -> [w752]
                      n352 = Subtract(x=3, y=w752) -> (x-y=w753:i32)
                      n353 = property on="Scope Graph" class="XYGraph (strict)"("Active Plot"=w753, "Plot.Visible?"=FALSE ("Plot.Visible")) -> ()  [unwired: 2 in, 2 out]
                    }
                    n354 = for {
                      N: w624 -> [_]
                      tunnel: [w749] -> w625 mode=indexing
                      i -> [w750]
                      n355 = property on="Scope Graph" class="XYGraph (strict)"("Active Plot"=w750) -> ("Plot.Visible?"=w749:bool)  [unwired: 2 in, 2 out]
                    }
                    n356 = Transpose 2D Array(2D array=w630) -> (transposed array=w629:string[][])
                    n357 = stacked-sequence {
                      seq-local: [_ w691 _ _] -> [_ _ w699 _]
                      tunnel: [w642 _ _ _] -> w633
                      tunnel: [w641 _ _ _] -> w623
                      tunnel: w631 -> [w640 _ _ _]
                      tunnel: w629 -> [w639 w693 w700 _]
                      tunnel: w626 -> [w638 _ _ _]
                      tunnel: w625 -> [w637 _ _ _]
                      tunnel: w624 -> [w636 w690 _ w737]
                      tunnel: w622 -> [w635 _ _ _]
                      frame #0 {
                        n358 = for {
                          N: w636 -> [_]
                          tunnel: [w656] -> w642 mode=indexing
                          tunnel: [w650] -> w641 mode=indexing
                          tunnel: w638 -> [w653] mode=indexing
                          tunnel: w640 -> [w655] mode=indexing
                          tunnel: w639 -> [w652] mode=indexing
                          tunnel: w637 -> [w648]
                          tunnel: w635 -> [w643]
                          i -> [w649]
                          n359 = for {
                            tunnel: w648 -> [w657] mode=indexing
                            tunnel: [w658] -> w647 if=w657
                            tunnel: [w657] -> w646
                            i -> [w658]
                            stop <- w657 stop-if-true
                          }
                          n360 = property on="Scope Graph" class="XYGraph (strict)"("Active Plot"=w649) -> ("Plot.Visible?"=w650:bool, "Plot.Plot Color"=w651:u32)  [unwired: 2 in, 2 out]
                          n361 = Select(t=w647, s=w646, f=-1) -> (s? t:f=w644:i32)
                          n362 = Not Equal?(x=w650, y=w653) -> (x != y?=w654:bool)
                          n363 = case shown="True" w650 {
                            tunnel: w651 -> [_ w660]
                            tunnel: w649 -> [_ w659]
                            frame False {
                            }
                            frame True {
                              n364 = Bundle(-1, w659) -> (w662:cluster{i32, i32})  [unwired: 1 in]
                              n365 = property on="Config Table" class="Tbl (strict)"("Active Cell"=w662, "CellFontColor"=w660) -> ()  [unwired: 2 in, 2 out]
                            }
                          }
                          n366 = case shown="True" w654 {
                            tunnel: [_ w666] -> w656
                            tunnel: w655 -> [_ w672]
                            tunnel: w652 -> [_ w684]
                            tunnel: w650 -> [_ w668]
                            tunnel: w649 -> [_ w675]
                            tunnel: w644 -> [_ w673]
                            tunnel: w643 -> [_ w664]
                            frame False {
                            }
                            frame True {
                              n367 = Index Array(array=w684) -> (element #1=w679:string, element #2=w680:string, element #3=w682:string, element #4=w683:string)  [unwired: 4 in]
                              n368 = case shown="False" w668 {
                                tunnel: w675 -> [_ w686]
                                tunnel: [w685 w686] -> w674
                                tunnel: w673 -> [w685 _]
                                frame False {
                                }
                                frame True {
                                }
                              }
                              n369 = Fract/Exp String To Number(string=w680) -> (number=w677:dbl)  [unwired: 3 in, 1 out]
                              n370 = Fract/Exp String To Number(string=w682) -> (number=w681:dbl)  [unwired: 3 in, 1 out]
                              n371 = Fract/Exp String To Number(string=w683) -> (number=w671:dbl)  [unwired: 3 in, 1 out]
                              n372 = case shown="\"GND\"" w679 {
                                tunnel: [w687 w688 w689] -> w667
                                frame "DC", Default {
                                w687 = 1 items=["AC", "DC", "GND"] ("vertical coupling (DC)")
                                }
                                frame "AC" {
                                w688 = 0 items=["AC", "DC", "GND"] ("vertical coupling (DC)")
                                }
                                frame "GND" {
                                w689 = 2 items=["AC", "DC", "GND"] ("vertical coupling (DC)")
                                }
                              }
                              n373 = local write "LastModGraph"(w674) -> ()
                              n374 = Multiply(x=8.0, y=w677) -> (x*y=w678:dbl)
                              n375 = node(w678) -> (w670:dbl[unit])
                              n376 = node(w681) -> (w669:dbl[unit])
                              n377 = Bundle("Substring"=w672, w671, w670, w669, "Plot.Visible?"=w668, "vertical coupling (DC)"=w667) -> (w665:T8)  [unwired: 1 in]
                              n378 = call "SendSetValue.vi"("Data"=w665, "PVName"="Configure_Channel_Msg", "PVConnections"=w664) -> ("error out"=w666:errorcluster)  [unwired: 7 in, 1 out]
                            }
                          }
                        }
                      }
                      frame #1 {
                        n379 = Transpose 2D Array(2D array=w693) -> (transposed array=w692:string[][])
                        n380 = Index Array(array=w692, index (row)=1 ("index")) -> (element=w697:string[])  [unwired: 1 in]
                        n381 = Array Subset(array=w697, length=w690) -> (w696:string[])  [unwired: 1 in]
                        n382 = Fract/Exp String To Number(string=w696) -> (number=w695:dbl[])  [unwired: 3 in, 1 out]
                        n383 = Array Max & Min(array=w695) -> (min value=w694:dbl)  [unwired: 3 out]
                        n384 = Divide(x=w694, y=w695) -> (x/y=w691:dbl[])
                        n385 = local write "Scaling-Array"(w691) -> ()
                      }
                      frame #2 {
                        n386 = local read "Time / DIV"() -> (w702:dbl[unit])
                        n387 = local read "Time/Record"() -> (w705:dbl)
                        n388 = local read "Complete\nData"() -> (w708:cluster{"Array":dbl[], "Y":dbl[]}[])
                        n389 = local read "Horizontal Offset"() -> (w701:dbl[unit])
                        n390 = local read "LastHorOffset"() -> (w710:dbl)
                        n391 = Multiply(x=w702, y=10.0) -> (x*y=w704:dbl[unit])
                        n392 = node(w704) -> (w706:dbl)
                        n393 = node(w701) -> (w709:dbl)
                        n394 = Divide(x=w705, y=w706) -> (x/y=w707:dbl)
                        n395 = for {
                          tunnel: w708 -> [w736] mode=indexing
                          tunnel: [w735] -> w711 mode=indexing
                          tunnel: w707 -> [w732]
                          tunnel: w710 -> [w727]
                          tunnel: w706 -> [w729]
                          tunnel: w709 -> [w726]
                          tunnel: w699 -> [w718] mode=indexing
                          tunnel: w700 -> [w714]
                          i -> [w713]
                          w730 = 500.0 ("y")
                          n396 = Unbundle(w736) -> ("Array"=w734:dbl[], "Y"=w717:dbl[])
                          n397 = Subtract(x=w734, y=w730) -> (x-y=w733:dbl[])
                          n398 = Subtract(x=w726, y=w727) -> (x-y=w728:dbl)
                          n399 = Index Array(array=w714, index (row)=w713, index (col)=2 ("index (row)")) -> (element=w716:string)
                          n400 = Multiply(x=w732, y=w733) -> (x*y=w731:dbl[])
                          n401 = Divide(x=w728, y=w729) -> (x/y=w725:dbl)
                          n402 = Fract/Exp String To Number(string=w716) -> (number=w715:dbl)  [unwired: 3 in, 1 out]
                          n403 = Add(x=w730, y=w731) -> (x+y=w723:dbl[])
                          n404 = Multiply(x=w725, y=1000.0) -> (x*y=w722:dbl)
                          n405 = Multiply(x=w718, y=w717) -> (x*y=w719:dbl[])
                          n406 = Add(x=w723, y=w722) -> (x+y=w721:dbl[])
                          n407 = Add(x=w715, y=w719) -> (x+y=w720:dbl[])
                          n408 = Bundle(w721, w720) -> (w735:cluster{dbl[], dbl[]})  [unwired: 1 in]
                        }
                        n409 = local write "Scope Graph"(w711) -> ()
                      }
                      frame #3 {
                        n410 = for {
                          N: w737 -> [_]
                          i -> [w739]
                          n411 = property on="Scope Graph" class="XYGraph (strict)"("Active Plot"=w739) -> ("Plot.Visible?"=w743:bool, "Plot.Plot Color"=w742:u32)  [unwired: 2 in, 2 out]
                          n412 = Add(x=4, y=w739) -> (x+y=w740:i32)
                          n413 = property on="Scope Graph" class="XYGraph (strict)"() -> ("AnntList"=w745:T2)  [unwired: 2 in, 2 out]
                          n414 = Select(t=w742, s=w743, f=u32 16777216) -> (s? t:f=w744:u32)
                          n415 = Index Array(array=w745, index=w740) -> (element=w747:T3)
                          n416 = Bundle By Name(cluster=w747, "Allow Drag"=w743, "Color"=w744) -> (w748:T3)
                          n417 = Replace Array Subset(array=w745, new element=w748, index=w740) -> (w746:T2)
                          n418 = property on="Scope Graph" class="XYGraph (strict)"("AnntList"=w746) -> ()  [unwired: 2 in, 2 out]
                        }
                      }
                    }
                    n419 = Merge Errors(w633) -> (w632:errorcluster)
                  }
                  event "RepeatButton": Value Change {
                    n420 = event-data() -> ("NewVal"=w759:bool)  [unwired: 1 in]
                    n421 = case shown="True" w759 {
                      tunnel: [_ w763] -> w758
                      tunnel: w755 -> [_ w761]
                      frame False {
                      }
                      frame True {
                        n422 = local write "Status LED"(u32 56387) -> ()
                        n423 = local read "Horizontal Scale"() -> (w764:i16)
                        n424 = call "SendSetValue.vi"("Data"=TRUE, "PVName"="Initiate_Acquisition_Msg", "PVConnections"=w761) -> ("error out"=w763:errorcluster)  [unwired: 7 in, 1 out]
                        n425 = local write "LHS"(w764) -> ()
                        n426 = local write "Start"(TRUE ("Start")) -> ()
                      }
                    }
                  }
                  event "One Button": Value Change {
                    n427 = event-data() -> ("NewVal"=w771:bool)  [unwired: 1 in]
                    n428 = case shown="True" w771 {
                      tunnel: [_ w777] -> w770
                      tunnel: w767 -> [_ w775]
                      frame False {
                      }
                      frame True {
                        n429 = local write "Status LED"(u32 56387) -> ()
                        n430 = local read "Horizontal Scale"() -> (w778:i16)
                        n431 = call "SendSetValue.vi"("Data"=TRUE ("Start"), "PVName"="Initiate_Acquisition_Msg", "PVConnections"=w775) -> ("error out"=w777:errorcluster)  [unwired: 7 in, 1 out]
                        n432 = local write "One Button"(FALSE ("Start")) -> ()
                        n433 = local write "Start"(TRUE ("Start")) -> ()
                        n434 = local write "LHS"(w778) -> ()
                      }
                    }
                  }
                  event "Config Table": Value Change {
                    n435 = event-data() -> ("OldVal"=w782:string[][], "NewVal"=w785:string[][])  [unwired: 1 in]
                    n436 = local read "Time / DIV"() -> (w798:dbl[unit])
                    n437 = local read "Time/Record"() -> (w801:dbl)
                    n438 = local read "Complete\nData"() -> (w795:cluster{"Array":dbl[], "Y":dbl[]}[])
                    n439 = local read "Horizontal Offset"() -> (w794:dbl[unit])
                    n440 = local read "LastHorOffset"() -> (w792:dbl)
                    n441 = Not Equal?(x=w782, y=w785) -> (x != y?=w807:bool[][])
                    n442 = Index Array(array=w785, index (row)=1 ("index")) -> (element=w790:string[])  [unwired: 1 in]
                    n443 = Multiply(x=w798, y=10.0) -> (x*y=w800:dbl[unit])
                    n444 = Array Subset(array=w790, length=w781) -> (w789:string[])  [unwired: 1 in]
                    n445 = node(w800) -> (w797:dbl)
                    n446 = node(w794) -> (w793:dbl)
                    n447 = Transpose 2D Array(2D array=w785) -> (transposed array=w784:string[][])
                    n448 = Transpose 2D Array(2D array=w807) -> (transposed array=w802:bool[][])
                    n449 = Fract/Exp String To Number(string=w789) -> (number=w788:dbl[])  [unwired: 3 in, 1 out]
                    n450 = Divide(x=w801, y=w797) -> (x/y=w796:dbl)
                    n451 = Array Max & Min(array=w788) -> (min value=w786:dbl)  [unwired: 3 out]
                    n452 = Divide(x=w786, y=w788) -> (x/y=w787:dbl[])
                    n453 = for {
                      tunnel: w784 -> [w823] mode=indexing
                      tunnel: w802 -> [w822] mode=indexing
                      tunnel: [w821] -> w805 mode=indexing
                      tunnel: w803 -> [w820] mode=indexing
                      tunnel: w783 -> [w817] mode=indexing
                      tunnel: w797 -> [w816]
                      tunnel: w796 -> [w815]
                      tunnel: w795 -> [w814]
                      tunnel: w793 -> [w813]
                      tunnel: w792 -> [w812]
                      tunnel: w787 -> [w811]
                      tunnel: w784 -> [w810]
                      tunnel: w783 -> [w809]
                      tunnel: w780 -> [w808]
                      n454 = Or Array Elements(Boolean array=w822) -> (logical OR=w819:bool)
                      n455 = case shown="True" w819 {
                        tunnel: [_ w836] -> w818
                        tunnel: w820 -> [_ w835]
                        tunnel: w823 -> [_ w833]
                        tunnel: w817 -> [_ w834]
                        tunnel: w816 -> [_ w832]
                        tunnel: w815 -> [_ w831]
                        tunnel: w814 -> [_ w830]
                        tunnel: w813 -> [_ w829]
                        tunnel: w812 -> [_ w828]
                        tunnel: w811 -> [_ w827]
                        tunnel: w810 -> [_ w826]
                        tunnel: w809 -> [_ w825]
                        tunnel: w808 -> [_ w824]
                        frame False {
                        }
                        frame True {
                          n456 = stacked-sequence {
                            seq-local: [_ _ _ _ w924 _] -> [_ _ _ _ _ w932]
                            seq-local: [_ _ _ w909 _ _] -> [_ _ _ _ w928 _]
                            tunnel: [w837 _ _ _ _ _] -> w836
                            tunnel: w835 -> [w846 _ _ _ _ _]
                            tunnel: w834 -> [w842 _ _ _ _ _]
                            tunnel: w833 -> [w850 _ _ _ _ _]
                            tunnel: w832 -> [_ w865 _ _ _ _]
                            tunnel: w831 -> [_ w864 _ _ _ _]
                            tunnel: w830 -> [_ w863 _ _ _ _]
                            tunnel: w829 -> [_ w862 _ _ _ _]
                            tunnel: w828 -> [_ w861 _ _ _ _]
                            tunnel: w827 -> [_ w860 _ _ w931 _]
                            tunnel: w826 -> [_ w859 w892 _ w930 _]
                            tunnel: w825 -> [_ _ w893 w910 _ _]
                            tunnel: w824 -> [w840 _ _ _ _ _]
                            frame #0 {
                              n457 = Index Array(array=w850) -> (element #1=w855:string, element #2=w854:string, element #3=w852:string, element #4=w851:string)  [unwired: 4 in]
                              n458 = Fract/Exp String To Number(string=w854) -> (number=w847:dbl)  [unwired: 3 in, 1 out]
                              n459 = Fract/Exp String To Number(string=w852) -> (number=w853:dbl)  [unwired: 3 in, 1 out]
                              n460 = Fract/Exp String To Number(string=w851) -> (number=w845:dbl)  [unwired: 3 in, 1 out]
                              n461 = case shown="\"DC\", Default" w855 {
                                tunnel: [w856 w857 w858] -> w841
                                frame "DC", Default {
                                w856 = 1 items=["AC", "DC", "GND"] ("vertical coupling (DC)")
                                }
                                frame "AC" {
                                w857 = 0 items=["AC", "DC", "GND"] ("vertical coupling (DC)")
                                }
                                frame "GND" {
                                w858 = 2 items=["AC", "DC", "GND"] ("vertical coupling (DC)")
                                }
                              }
                              n462 = Multiply(x=8.0, y=w847) -> (x*y=w849:dbl)
                              n463 = node(w849) -> (w844:dbl[unit])
                              n464 = node(w853) -> (w843:dbl[unit])
                              n465 = Bundle("Substring"=w846, w845, w844, w843, "Plot.Visible?"=w842, "vertical coupling (DC)"=w841) -> (w839:T8)  [unwired: 1 in]
                              n466 = call "SendSetValue.vi"("Data"=w839, "PVName"="Configure_Channel_Msg", "PVConnections"=w840) -> ("error out"=w837:errorcluster)  [unwired: 7 in, 1 out]
                            }
                            frame #1 {
                              n467 = for {
                                tunnel: w863 -> [w891] mode=indexing
                                tunnel: [w890] -> w866 mode=indexing
                                tunnel: w864 -> [w887]
                                tunnel: w861 -> [w882]
                                tunnel: w865 -> [w884]
                                tunnel: w862 -> [w881]
                                tunnel: w860 -> [w873] mode=indexing
                                tunnel: w859 -> [w869]
                                i -> [w868]
                                w885 = 500.0 ("y")
                                n468 = Unbundle(w891) -> ("Array"=w889:dbl[], "Y"=w872:dbl[])
                                n469 = Subtract(x=w889, y=w885) -> (x-y=w888:dbl[])
                                n470 = Subtract(x=w881, y=w882) -> (x-y=w883:dbl)
                                n471 = Index Array(array=w869, index (row)=w868, index (col)=2 ("index (row)")) -> (element=w871:string)
                                n472 = Multiply(x=w887, y=w888) -> (x*y=w886:dbl[])
                                n473 = Divide(x=w883, y=w884) -> (x/y=w880:dbl)
                                n474 = Fract/Exp String To Number(string=w871) -> (number=w870:dbl)  [unwired: 3 in, 1 out]
                                n475 = Add(x=w885, y=w886) -> (x+y=w878:dbl[])
                                n476 = Multiply(x=w880, y=1000.0) -> (x*y=w877:dbl)
                                n477 = Multiply(x=w873, y=w872) -> (x*y=w874:dbl[])
                                n478 = Add(x=w878, y=w877) -> (x+y=w876:dbl[])
                                n479 = Add(x=w870, y=w874) -> (x+y=w875:dbl[])
                                n480 = Bundle(w876, w875) -> (w890:cluster{dbl[], dbl[]})  [unwired: 1 in]
                              }
                              n481 = local write "Scope Graph"(w866) -> ()
                            }
                            frame #2 {
                              n482 = for {
                                tunnel: w893 -> [w903] mode=indexing
                                tunnel: w892 -> [w897]
                                i -> [w896]
                                n483 = property on="Scope Graph" class="XYGraph (strict)"("Active Plot"=w896) -> ("AnntList"=w906:T2, "Plot.Plot Color"=w904:u32)  [unwired: 2 in, 2 out]
                                n484 = Index Array(array=w897, index (row)=w896, index (col)=2 ("index (row)")) -> (element=w901:string)
                                n485 = Add(x=w896, y=4) -> (x+y=w895:i32)
                                n486 = Fract/Exp String To Number(string=w901) -> (number=w899:dbl)  [unwired: 3 in, 1 out]
                                n487 = Select(t=w904, s=w903, f=u32 16777216) -> (s? t:f=w898:u32)
                                n488 = Index Array(array=w906, index=w895) -> (element=w905:T3)
                                n489 = Bundle By Name(cluster=w905, "Color"=w898, "Position.Y"=w899) -> (w908:T3)
                                n490 = Replace Array Subset(array=w906, new element=w908, index=w895) -> (w907:T2)
                                n491 = property on="Scope Graph" class="XYGraph (strict)"("AnntList"=w907) -> ()  [unwired: 2 in, 2 out]
                              }
                            }
                            frame #3 {
                              n492 = local read "LastModGraph"() -> (w916:i8)
                              n493 = Array Subset(array=w910, length=w916) -> (w918:bool[])  [unwired: 1 in]
                              n494 = Index Array(array=w910, index=w916) -> (element=w919:bool)
                              n495 = Reverse 1D Array(array=w918) -> (reversed array=w917:bool[])
                              n496 = for {
                                tunnel: w917 -> [w920] mode=indexing
                                tunnel: [w921] -> w912
                                tunnel: [w920] -> w915
                                i -> [w921]
                                stop <- w920 stop-if-true
                              }
                              n497 = Decrement(x=w912) -> (x-1=w913:i32)
                              n498 = Select(t=w912, s=w915, f=w913) -> (s? t:f=w914:i32)
                              n499 = Subtract(x=w916, y=w914) -> (x-y=w911:i32)
                              n500 = Select(t=w916, s=w919, f=w911) -> (s? t:f=w909:i32)
                            }
                            frame #4 {
                              n501 = Index Array(array=w930, index (row)=w928, index (col)=2 ("index (row)")) -> (element=w929:string)
                              n502 = Fract/Exp String To Number(string=w929) -> (number=w922:dbl)  [unwired: 3 in, 1 out]
                              n503 = local read "OrigCursPosVer"() -> (w923:dbl[])
                              n504 = Index Array(array=w931, index=w928) -> (element=w926:dbl)
                              n505 = Multiply(x=w926, y=w923) -> (x*y=w925:dbl[])
                              n506 = Add(x=w925, y=w922) -> (x+y=w924:dbl[])
                            }
                            frame #5 {
                              n507 = for {
                                tunnel: i32[] [2, 3] -> [w935] mode=indexing
                                tunnel: w932 -> [w934] mode=indexing
                                n508 = property on="Scope Graph" class="XYGraph (strict)"() -> ("AnntList"=w939:T2)  [unwired: 2 in, 2 out]
                                n509 = Index Array(array=w939, index=w935) -> (element=w937:T3)
                                n510 = Bundle By Name(cluster=w937, "Position.Y"=w934) -> (w936:T3)
                                n511 = Replace Array Subset(array=w939, new element=w936, index=w935) -> (w938:T2)
                                n512 = property on="Scope Graph" class="XYGraph (strict)"("AnntList"=w938) -> ()  [unwired: 2 in, 2 out]
                              }
                            }
                          }
                        }
                      }
                      n513 = Merge Errors(w818) -> (w821:errorcluster)
                    }
                    n514 = local write "Scaling-Array"(w787) -> ()
                    n515 = Merge Errors(w805) -> (w804:errorcluster)
                  }
                  event "Scope Graph": Cursor Move {
                    n516 = event-data() -> ("CursIdx"=w942:i32, "CursLoc"=w941:cluster{"X":dbl, "Y":dbl})  [unwired: 1 in]
                    n517 = stacked-sequence {
                      seq-local: [w945 _] -> [_ w960]
                      seq-local: [w944 _] -> [_ w961]
                      tunnel: w942 -> [_ w959]
                      tunnel: w941 -> [_ w958]
                      tunnel: w940 -> [w954 _]
                      frame #0 {
                        # "Take the last activated graph, or if a graph was deactivated\ntake the previous one"
                        n518 = local read "LastModGraph"() -> (w951:i8)
                        n519 = Array Subset(array=w954, length=w951) -> (w953:bool[])  [unwired: 1 in]
                        n520 = Index Array(array=w954, index=w951) -> (element=w955:bool)
                        n521 = Reverse 1D Array(array=w953) -> (reversed array=w952:bool[])
                        n522 = for {
                          tunnel: w952 -> [w956] mode=indexing
                          tunnel: [w957] -> w947
                          tunnel: [w956] -> w950
                          i -> [w957]
                          stop <- w956 stop-if-true
                        }
                        n523 = Decrement(x=w947) -> (x-1=w948:i32)
                        n524 = Select(t=w947, s=w950, f=w948) -> (s? t:f=w949:i32)
                        n525 = Subtract(x=w951, y=w949) -> (x-y=w946:i32)
                        n526 = Select(t=w951, s=w955, f=w946) -> (s? t:f=w945:i32)
                        n527 = Less Than 0?(x=w945) -> (x < 0?=w944:bool)
                      }
                      frame #1 {
                        n528 = case shown="False" w961 {
                          tunnel: w958 -> [w964 _]
                          tunnel: w959 -> [w963 _]
                          tunnel: w960 -> [w962 _]
                          frame False {
                            n529 = case shown="Default" w963 {
                              tunnel: w964 -> [w978 w1001 w1025 w1050 _]
                              tunnel: w962 -> [_ _ w1017 w1042 _]
                              frame 0 {
                                w983 = 10
                                n530 = local read "Time / DIV"() -> (w977:dbl[unit])
                                n531 = Unbundle By Name(w978) -> ("X"=w974:dbl)
                                n532 = local read "Horizontal Offset"() -> (w968:dbl[unit])
                                n533 = node(w977) -> (w972:dbl)
                                n534 = Multiply(x=w972, y=5.0) -> (x*y=w971:dbl)
                                n535 = Divide(x=w972, y=100.0) -> (x/y=w975:dbl)
                                n536 = node(w968) -> (w967:dbl)
                                n537 = Multiply(x=w975, y=w974) -> (x*y=w970:dbl)
                                n538 = Subtract(x=w970, y=w971) -> (x-y=w969:dbl)
                                n539 = property on="Scope Graph" class="XYGraph (strict)"() -> ("YScale.Maximum"=w982:dbl)  [unwired: 2 in, 2 out]
                                n540 = Add(x=w969, y=w967) -> (x+y=w965:dbl)
                                n541 = local write "OrgCurPosLeft"(w965) -> ()
                                n542 = call "CalcTimeLabel.vi"("InputTime"=w965) -> ("TimeString"=w966:string)
                                n543 = Multiply(x=w982, y=0.95) -> (x*y=w981:dbl)
                                n544 = property on="Scope Graph" class="XYGraph (strict)"() -> ("AnntList"=w986:T2)  [unwired: 2 in, 2 out]
                                n545 = Index Array(array=w986, index=w983) -> (element=w985:T3)
                                n546 = Bundle By Name(cluster=w985, "Name"=w966, "Label Offset.Y"=w981, "Name Visible"=TRUE) -> (w984:T3)
                                n547 = Replace Array Subset(array=w986, new element=w984, index=w983) -> (w987:T2)
                                n548 = property on="Scope Graph" class="XYGraph (strict)"("AnntList"=w987) -> ()  [unwired: 2 in, 2 out]
                              }
                              frame 1 {
                                w1006 = 11
                                n549 = local read "Time / DIV"() -> (w1000:dbl[unit])
                                n550 = Unbundle By Name(w1001) -> ("X"=w997:dbl)
                                n551 = local read "Horizontal Offset"() -> (w991:dbl[unit])
                                n552 = node(w1000) -> (w995:dbl)
                                n553 = Multiply(x=w995, y=5.0) -> (x*y=w994:dbl)
                                n554 = Divide(x=w995, y=100.0) -> (x/y=w998:dbl)
                                n555 = node(w991) -> (w990:dbl)
                                n556 = Multiply(x=w998, y=w997) -> (x*y=w993:dbl)
                                n557 = Subtract(x=w993, y=w994) -> (x-y=w992:dbl)
                                n558 = property on="Scope Graph" class="XYGraph (strict)"() -> ("YScale.Maximum"=w1005:dbl)  [unwired: 2 in, 2 out]
                                n559 = Add(x=w992, y=w990) -> (x+y=w988:dbl)
                                n560 = local write "OrgCurPosRight"(w988) -> ()
                                n561 = call "CalcTimeLabel.vi"("InputTime"=w988) -> ("TimeString"=w989:string)
                                n562 = Multiply(x=w1005, y=0.87) -> (x*y=w1004:dbl)
                                n563 = property on="Scope Graph" class="XYGraph (strict)"() -> ("AnntList"=w1009:T2)  [unwired: 2 in, 2 out]
                                n564 = Index Array(array=w1009, index=w1006) -> (element=w1008:T3)
                                n565 = Bundle By Name(cluster=w1008, "Name"=w989, "Label Offset.Y"=w1004, "Name Visible"=TRUE) -> (w1007:T3)
                                n566 = Replace Array Subset(array=w1009, new element=w1007, index=w1006) -> (w1010:T2)
                                n567 = property on="Scope Graph" class="XYGraph (strict)"("AnntList"=w1010) -> ()  [unwired: 2 in, 2 out]
                              }
                              frame 2 {
                                w1031 = 9
                                n568 = local read "Config Table"() -> (w1023:string[][])
                                n569 = local read "OrigCursPosVer"() -> (w1013:dbl[])
                                n570 = local read "Scaling-Array"() -> (w1018:dbl[])
                                n571 = Unbundle By Name(w1025) -> ("Y"=w1019:dbl)
                                n572 = Index Array(array=w1023, index (row)=2, index (col)=w1017) -> (element=w1024:string)
                                n573 = Index Array(array=w1018, index=w1017) -> (element=w1015:dbl)
                                n574 = property on="Scope Graph" class="XYGraph (strict)"("Active Plot"=w1017) -> ("Plot.Plot Color"=w1026:u32)  [unwired: 2 in, 2 out]
                                n575 = Fract/Exp String To Number(string=w1024) -> (number=w1021:dbl)  [unwired: 3 in, 1 out]
                                n576 = Subtract(x=w1019, y=w1021) -> (x-y=w1016:dbl)
                                n577 = Divide(x=w1016, y=w1015) -> (x/y=w1011:dbl)
                                n578 = Replace Array Subset(array=w1013, new element=w1011, index=0) -> (w1014:dbl[])
                                n579 = local write "OrigCursPosVer"(w1014) -> ()
                                n580 = property on="Scope Graph" class="XYGraph (strict)"() -> ("AnntList"=w1034:T2)  [unwired: 2 in, 2 out]
                                n581 = property on="Scope Graph" class="XYGraph (strict)"() -> ("YScale.Maximum"=w1030:dbl)  [unwired: 2 in, 2 out]
                                n582 = Index Array(array=w1034, index=w1031) -> (element=w1033:T3)
                                n583 = call "CalcVoltLabel.vi"("InputVolt"=w1011) -> ("VoltString"=w1020:string)
                                n584 = Multiply(x=w1030, y=0.95) -> (x*y=w1029:dbl)
                                n585 = Bundle By Name(cluster=w1033, "Name"=w1020, "Label Offset.Y"=w1029, "Name Visible"=TRUE, "Color"=w1026) -> (w1032:T3)
                                n586 = Replace Array Subset(array=w1034, new element=w1032, index=w1031) -> (w1035:T2)
                                n587 = property on="Scope Graph" class="XYGraph (strict)"("AnntList"=w1035) -> ()  [unwired: 2 in, 2 out]
                              }
                              frame 3 {
                                w1056 = 8
                                n588 = local read "Config Table"() -> (w1048:string[][])
                                n589 = local read "OrigCursPosVer"() -> (w1038:dbl[])
                                n590 = local read "Scaling-Array"() -> (w1043:dbl[])
                                n591 = Unbundle By Name(w1050) -> ("Y"=w1044:dbl)
                                n592 = Index Array(array=w1048, index (row)=2, index (col)=w1042) -> (element=w1049:string)
                                n593 = Index Array(array=w1043, index=w1042) -> (element=w1040:dbl)
                                n594 = property on="Scope Graph" class="XYGraph (strict)"("Active Plot"=w1042) -> ("Plot.Plot Color"=w1051:u32)  [unwired: 2 in, 2 out]
                                n595 = Fract/Exp String To Number(string=w1049) -> (number=w1046:dbl)  [unwired: 3 in, 1 out]
                                n596 = Subtract(x=w1044, y=w1046) -> (x-y=w1041:dbl)
                                n597 = Divide(x=w1041, y=w1040) -> (x/y=w1036:dbl)
                                n598 = Replace Array Subset(array=w1038, new element=w1036, index=1) -> (w1039:dbl[])
                                n599 = local write "OrigCursPosVer"(w1039) -> ()
                                n600 = property on="Scope Graph" class="XYGraph (strict)"() -> ("AnntList"=w1059:T2)  [unwired: 2 in, 2 out]
                                n601 = property on="Scope Graph" class="XYGraph (strict)"() -> ("YScale.Maximum"=w1055:dbl)  [unwired: 2 in, 2 out]
                                n602 = Index Array(array=w1059, index=w1056) -> (element=w1058:T3)
                                n603 = call "CalcVoltLabel.vi"("InputVolt"=w1036) -> ("VoltString"=w1045:string)
                                n604 = Multiply(x=w1055, y=0.87) -> (x*y=w1054:dbl)
                                n605 = Bundle By Name(cluster=w1058, "Name"=w1045, "Label Offset.Y"=w1054, "Name Visible"=TRUE, "Color"=w1051) -> (w1057:T3)
                                n606 = Replace Array Subset(array=w1059, new element=w1057, index=w1056) -> (w1060:T2)
                                n607 = property on="Scope Graph" class="XYGraph (strict)"("AnntList"=w1060) -> ()  [unwired: 2 in, 2 out]
                              }
                              frame Default {
                              }
                            }
                          }
                          frame True {
                          }
                        }
                      }
                    }
                  }
                  event "Scope Graph": Mouse Down? {
                    # "It is not possible to switch off the shortcut menu within the graph\non cursors in another way. This is not nice since it also means that\nno other runtime menu can be implemented..."
                    n608 = event-data() -> ("Button"=w1063:u16)  [unwired: 1 in, 7 out]
                    n609 = Equal?(x=w1063, y=u16 2) -> (x = y?=w1061:bool)
                    n610 = event-data("Discard?"=w1061) -> ()  [unwired: 1 in, 1 out]
                  }
                  event Menu Selection (User) {
                    n611 = event-data() -> ("ItemTag"=w1068:string)  [unwired: 1 in]
                    n612 = case shown="\"SAVE\"" w1068 {
                      tunnel: [_ TRUE _] -> w1067
                      tunnel: w1066 -> [_ _ w1085]
                      frame Default {
                      }
                      frame "QUIT" {
                      }
                      frame "SAVE" {
                        # "The idea here is that the original data is stored independent\nof what is actually displayed in the graph. For the offset this\nmeans that only the offset value sent to the device matters."
                        n613 = local read "Complete\nData"() -> (w1079:cluster{"Array":dbl[], "Y":dbl[]}[])
                        n614 = local read "Time/Record"() -> (w1077:dbl)
                        n615 = local read "LastHorOffset"() -> (w1072:dbl)
                        n616 = Index Array(array=w1079) -> (element=w1084:cluster{"Array":dbl[], "Y":dbl[]})  [unwired: 1 in]
                        n617 = Unbundle(w1084) -> ("Array"=w1087:dbl[])  [unwired: 1 out]
                        n618 = Subtract(x=w1087, y=500 ("Numeric Control")) -> (x-y=w1076:dbl[])
                        n619 = for {
                          N: w1085 -> [_]
                          tunnel: w1079 -> [w1092] mode=indexing
                          tunnel: [w1091] -> w1082 mode=indexing
                          n620 = Unbundle(w1092) -> ("Y"=w1091:dbl[])  [unwired: 1 out]
                        }
                        n621 = Multiply(x=w1076, y=w1077) -> (x*y=w1086:dbl[])
                        n622 = Divide(x=w1086, y=1000 ("Numeric Control")) -> (x/y=w1074:dbl[])
                        n623 = Transpose 2D Array(2D array=w1082) -> (transposed array=w1081:dbl[][])
                        n624 = Add(x=w1074, y=w1072) -> (x+y=w1083:dbl[])
                        n625 = for {
                          tunnel: w1083 -> [w1090] mode=indexing
                          tunnel: w1081 -> [w1089] mode=indexing
                          tunnel: [w1088] -> w1080 mode=indexing
                          n626 = Build Array (concatenate)(w1090, w1089) -> (w1088:dbl[])
                        }
                        n627 = call-poly <vilib>:"Write To Spreadsheet File.vi"("format (%.3f)"="%.3e", "2D data"=w1080) -> ()  [unwired: 6 in, 1 out]
                      }
                    }
                  }
                  event User Event {
                    n628 = event-data() -> ("Stop"=w1094:bool)  [unwired: 1 in]
                    n629 = local write "Abort Button"(w1094) -> ()
                  }
                  event "Abort Button": Value Change {
                    n630 = event-data() -> ("NewVal"=w1096:bool)  [unwired: 1 in]
                    n631 = case shown="True" w1096 {
                      tunnel: w1098 -> [_ w1103]
                      tunnel: [_ w1102] -> w1097
                      frame False {
                      }
                      frame True {
                        n632 = local write "Abort Button"(FALSE ("Abort Button")) -> ()
                        n633 = call "SendSetValue.vi"("Data"=TRUE, "PVName"="Abort_Msg", "PVConnections"=w1103) -> ("error out"=w1102:errorcluster)  [unwired: 7 in, 1 out]
                      }
                    }
                  }
                  event Panel Close? {
                    n634 = event-data() -> ()  [unwired: 1 in, 1 out]
                    n635 = call <vilib>:"Read Self Enqueuer.vi"("Actor"=w1109) -> ("Self Enqueuer"=w1111:refnum<class "Message Enqueuer.lvclass">)  [unwired: 10 in]
                    n636 = local write "Abort Button"(TRUE ("Stop Button")) -> ()
                    n637 = call <vilib>:"Send Normal Stop.vi"("Message Enqueuer"=w1111) -> ("error out"=w1110:errorcluster)  [unwired: 10 in]
                    n638 = call <vilib>:"Simple Error Handler.vi"("error in (no error)"=w1110) -> ()  [unwired: 4 in, 5 out]
                    n639 = event-data("Discard?"=TRUE) -> ()  [unwired: 1 in, 1 out]
                  }
                }
                n640 = call <vilib>:"Simple Error Handler.vi"("error in (no error)"=w245) -> ()  [unwired: 4 in, 5 out]
              }
              n641 = Unregister For Events(event registration refnum=w234) -> (error out=w233:errorcluster)  [unwired: 1 in]
              n642 = call-dynamic "Destroy User Define Events.vi"("error in (no error)"=w233, "CS++GUIActor in"=w231) -> ()  [unwired: 8 in, 2 out]
            }
            frame #8 {
              # "ToDo: This destroys the complete device object.\nMaybe someone only wants to close the GUI. \nBut in this case one should also be able to only \nopen the GUI without starting a second Proxy which\nwill not work (--> Object Manager)"
              n643 = for {
                tunnel: w1115 -> [w1127] mode=indexing
                n644 = call "Disconnect.vi"("PVConnection in"=w1127) -> ()  [unwired: 9 in, 2 out]
              }
              n645 = call "Open Actor Core FP.vi"("Open FP (F)"=FALSE, "CS++BaseActor in"=w1117) -> ("error out"=w1113:errorcluster, "CS++BaseActor out"=w1114:refnum<class "CS++ScopeGui.lvclass">)  [unwired: 8 in]
              n646 = disable-structure shown="Enabled" {
                disable-tunnel: w1114 -> [w1122 _]
                disable-tunnel: w1113 -> [w1120 _]
                frame Enabled {
                  n647 = property class="CS++ScopeGui.lvclass"(reference=w1122, error in=w1120) -> (error out=w1121:errorcluster, "Accessors:Associated Proxy Actor Enqueuer"=w1119:refnum<class "Message Enqueuer.lvclass">)  [unwired: 1 out]
                  n648 = call <vilib>:"Equals Not A Refnum.vi"("Message Enqueuer"=w1119) -> ("Not a refnum?"=w1118:bool)  [unwired: 10 in]
                  n649 = case shown="False" w1118 {
                    tunnel: [w1125 w1126] -> _
                    tunnel: w1119 -> [w1124 _]
                    tunnel: w1121 -> [w1123 w1126]
                    frame False {
                      n650 = call <vilib>:"Send Normal Stop.vi"("error in (no error)"=w1123, "Message Enqueuer"=w1124) -> ("error out"=w1125:errorcluster)  [unwired: 9 in]
                    }
                    frame True {
                    }
                  }
                }
                frame Disabled {
                }
              }
            }
          }
        }
        frame Error {
        }
      }
    }
  }
  n651 = call-parent "Actor Core.vi"("error in"=w5, "CS++DeviceGUIActor.lvclass"=w6) -> ("Error Out"=→"Error Out":errorcluster, "Actor out"=→"Actor out":refnum<class "Actor.lvclass">)  [unwired: 8 in]
